vi "SCA-RT_old.vi"() -> ()   [LabVIEW 2016]
uses:
  <vilib>/Platform/TimedLoop/XDataNode/wakeup.ctl
  <vilib>/Platform/TimedLoop/XDataNode/XDNodeRunTimeDep.lvlib
  <vilib>/Platform/TimedLoop/XDataNode/nitl_modes.ctl
  <vilib>/Platform/TimedLoop/XDataNode/timing_clust.ctl
  <vilib>/Platform/TimedLoop/XDataNode/XDataNode.xnode
  <vilib>/Motion/BlockNode/FB.NIMotion.xnode
  <vilib>/Platform/TimedLoop/XDataNode/loadnilvce.vi
  Users/wymanm/Desktop/Sample Changer - Copy/controls/state control sample changer.ctl
  <vilib>/Instr/_visa.llb/VISA Configure Serial Port (Instr).vi
  <vilib>/Analysis/NI_AALBase.lvlib
  <vilib>/Analysis/baseanly.llb/Mean (DBL).vi
  controls/SCA states.ctl
  controls/Encoder bit cluster.ctl
  Common-Control/Gate Valve Readback.ctl
  Common-Control/Horizontal Rod states.ctl
  controls/Vertical Rod states.ctl
  <vilib>/NI_Real-Time Target Support.lvlib
  <vilib>/Motion/Express/_s/nimc.fb.straightLineMove.startStraightLineMove.axis.modeRelative.0.vi
  Common-Control/GP307 cluster.ctl
panel:
  in  "Sample Rod Min Count":u32
  in  "Sample Rod Max Count":u32
  in  "Insert Rod Max Count":u32
  in  "Insert Rod Min Count":u32
  in  "Retract Rod Min Count":u32
  in  "Retract Rod Max Count":u32
  out "Encoder loop error":errorcluster
  out "Convectron readback loop error":errorcluster
  out "HV Control loop error":errorcluster
  out "Rotate Wheel error":errorcluster
  out "Ion Source Vac Cluster":T1
  out "Bellows Vac Cluster":T1
  in  "Wheel GV Min Count":i32
  out "Start Sample Change":bool
  out "SCA-cRIO error":errorcluster
  in  "Rollover Sample":i8=54
  out "Insert Rod Status":T2
  out "Retract Rod Status":T2
  out "Sample Rod status":T3
  out "Wheel GV":T4
  out "Raw bits":bool[](array[boolean])
  out "Converted bits":bool[](array[boolean])
  out "Immersion Lens I read":dbl format="%0.2f"
  out "Immersion Lens V read":dbl format="%0.2f"
  out "SCA next state":T5
  out "Extractor I read":dbl
  out "Extractor V read":dbl
  out "Extractor V set":dbl
  out "Cathode V read":dbl
  out "Cathode I read":dbl
  out "Cathode V set":dbl
  in  "Execute Move":bool
  out "New Move":dbl
  out "Encoder Destination":dbl
  in  "Step Window Radius":i16=2
  out "In Range?":bool
  out "Window Limit 2":u32
  out "Window Limit 1":u32
  out "Encoder position":u16
  out "change sample start end":bool
  out "start sample change":bool
  in  "clear error 3":bool
  in  "clear error 2":bool
  out "set cold cathode on 2":bool
  out "Rotate Wheel":bool
  out "Venting Source":bool
  out "Pumping out Source":bool
  out "insert Retract Rod":bool
  out "retract Retract Rod":bool
  out "Open Wheel GV":bool
  out "Close Wheel GV":bool
  out "insert Insert Rod":bool
  out "retract Insert Rod":bool
  out "insert Sample Rod":bool
  out "retract Sample Rod":bool
  in  "clear error":bool
  out "action":string
  out "Vac Readback Loop error":errorcluster
  out "Sample Wheel Convectron":string
  out "Sample Rod UP sensor":bool
  out "Sample Rod DOWN sensor":bool
  out "done":bool
  out "Insert Rod IN sensor":bool
  out "Insert Rod OUT sensor":bool
  out "Retract Rod IN sensor":bool
  out "Retract Rod OUT sensor":bool
  out "Sensor loop error":errorcluster
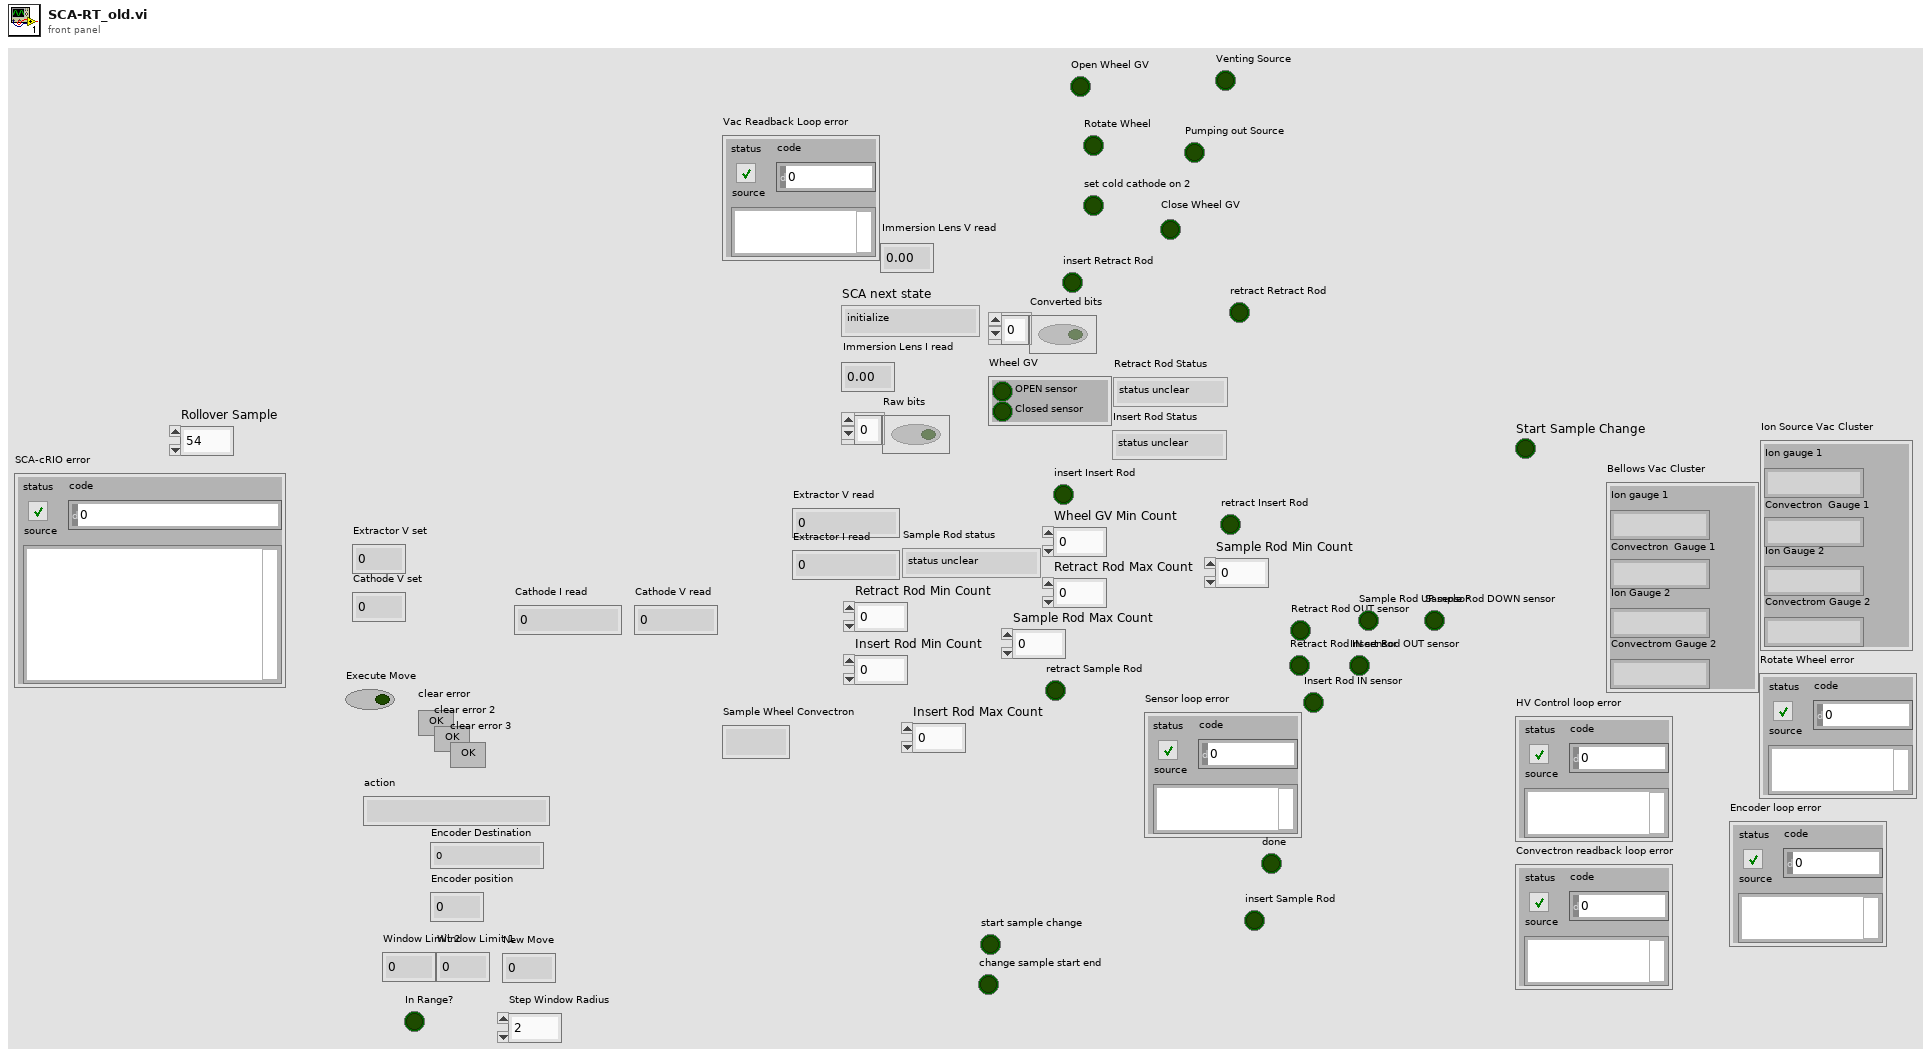
[diagram p1: front panel]
types:
  T1 = typedef "GP307 cluster.ctl" = cluster{"Ion gauge 1":string, "Convectron  Gauge 1 ":string, "Ion Gauge 2":string, "Convectrom Gauge 2":string}
  T2 = typedef "Horizontal Rod states.ctl" = enum16{"status unclear", "rod in", "rod out"}
  T3 = typedef "Vertical Rod states.ctl" = enum16{"status unclear", "rod down", "rod up"}
  T4 = typedef "Gate Valve Readback.ctl" = cluster{"OPEN sensor":bool, "Closed sensor":bool}
  T5 = typedef "SCA states.ctl" = enum16{"initialize", "wait", "change sample start", "change sample", "check position", "wait position", "rotate wheel", "sample change complete", "sample rod up", "sample rod down", "retract rod in", "retract rod out", "insert rod in", "insert rod out", "wheel GV open", "wheel GV close", "vent source", "pump source"}
  T6 = typedef "GV states.ctl" = enum16{"status unclear", "closed", "open"}
  T7 = typedef "XDNodeRunTimeDep.lvlib/timing_clust.ctl" = cluster{"Expected End [f-1]":u64, "Actual End [f-1]":u64, "Finished Late? [f-1]":bool, "Expected End [i-1]":u64, "Actual End [i-1]":u64, "Finished Late? [i-1]":bool, "Expected Start [i]":u64, "Actual Start [i]":u64, "Expected Start [f]":u64, "Actual Start [f]":u64, "Source Name":string, "Structure Name":string, "Period":i64, "Deadline":i64, "Offset":i64, "Start":i64, "Priority":i32, "Timeout":i32, "Mode":T8, "Wakeup Reason":T9, "Error":errorcluster, "Source Type":string, "Secondary Source Type":string, "Global End Time":u64, "Global Start Time":u64, "Frame Duration":u64, "Iteration Duration":u64, "Assigned CPU":i32, "I/O Scan Engine Mode":u32}
  T8 = typedef "XDNodeRunTimeDep.lvlib/nitl_modes.ctl" = enum32{"No Change", "Process missed periods, maintain original phase", "Discard missed periods, maintain original phase", "Process missed periods, ignore original phase", "Discard missed periods, ignore original phase"}
  T9 = typedef "XDNodeRunTimeDep.lvlib/wakeup.ctl" = enum32{"Normal", "Aborted", "Asynchronous wakeup", "Timing source error", "Timed loop error", "Timeout"}
  T10 = typedef "Encoder bit cluster.ctl" = cluster{"MSB":bool, "13th bit":bool, "12th bit":bool, "11th bit":bool, "10th bit":bool, "9th bit":bool, "8th bit":bool, "7th bit":bool, "6th bit":bool, "5th bit":bool, "4th bit":bool, "3rd bit":bool, "2nd bit":bool, "LSB":bool}
  T11 = typedef "state control sample changer.ctl" = string
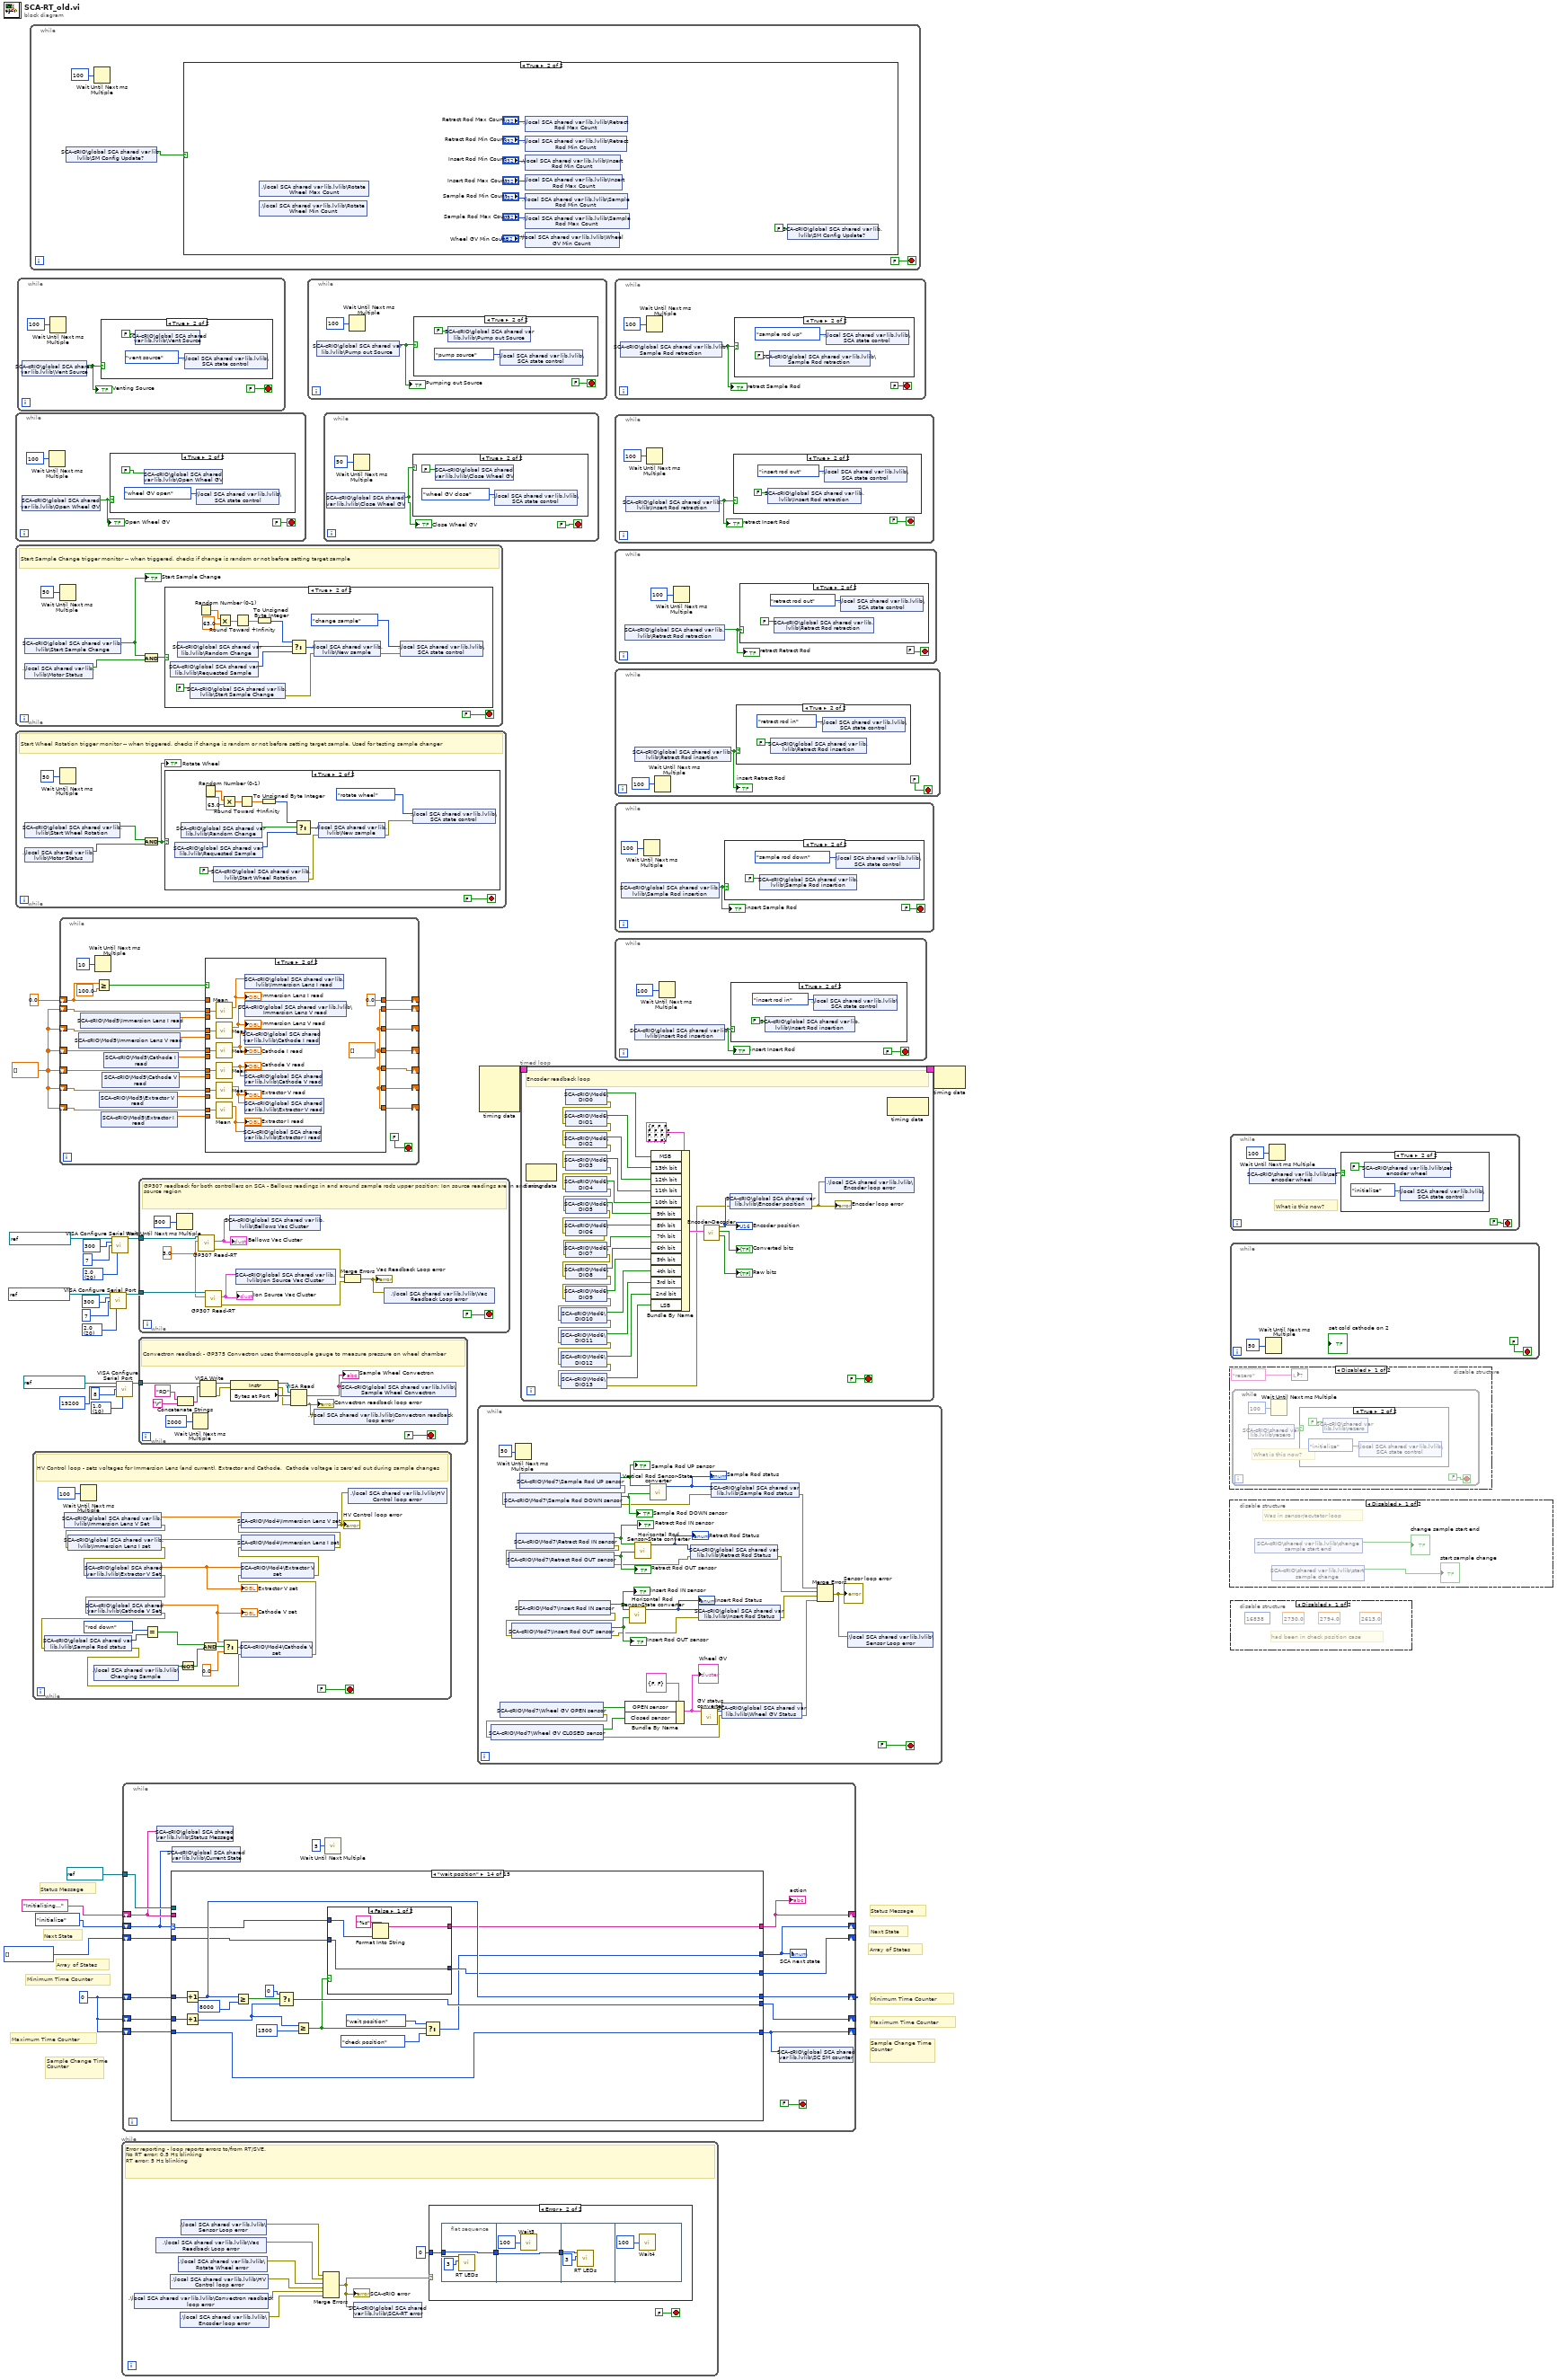
[diagram p0: block diagram]
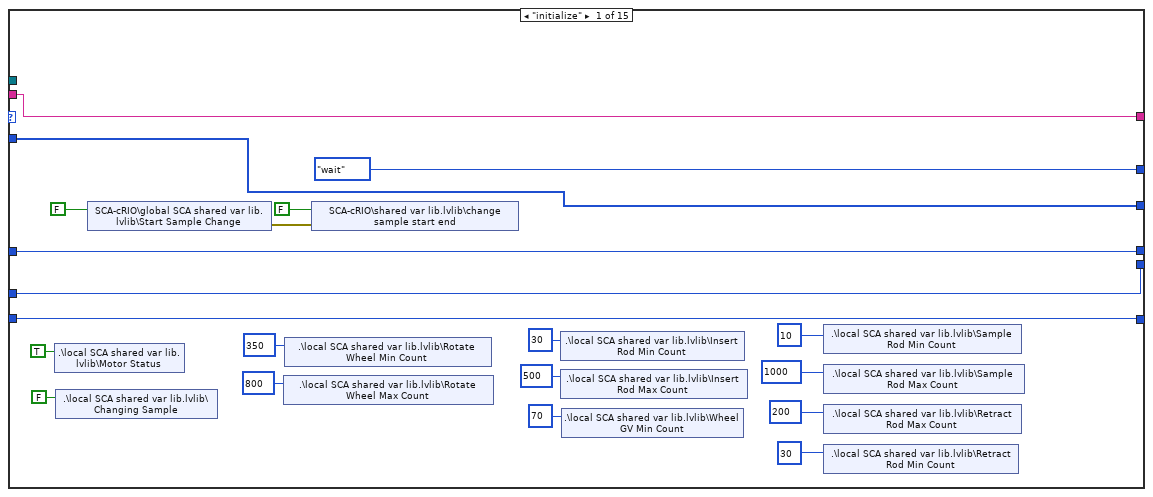
[diagram p5: hidden frame]
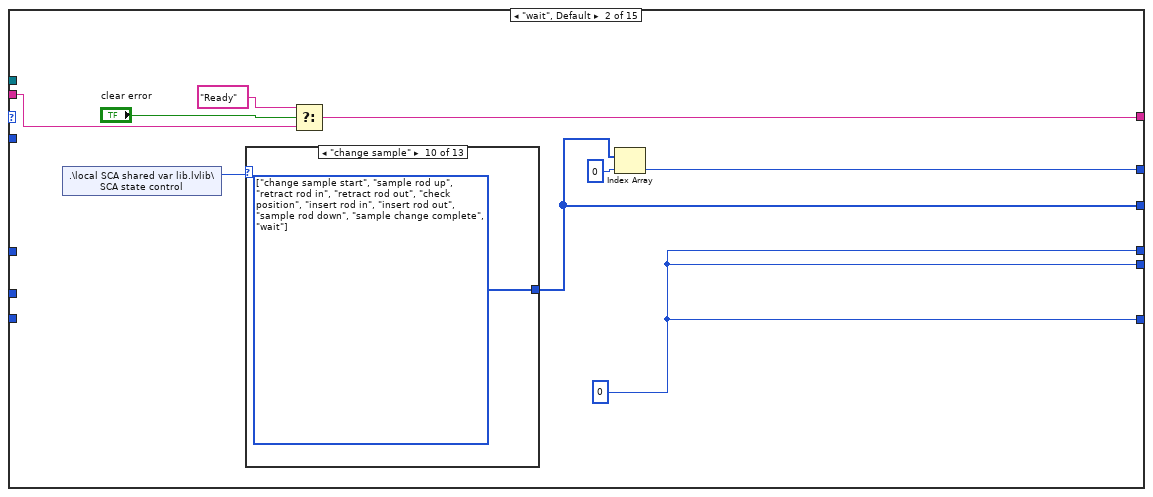
[diagram p6: hidden frame]
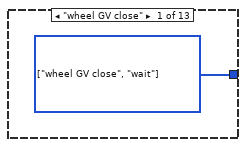
[diagram p7: hidden frame]
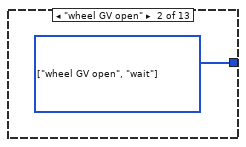
[diagram p8: hidden frame]
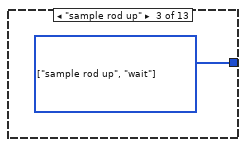
[diagram p9: hidden frame]
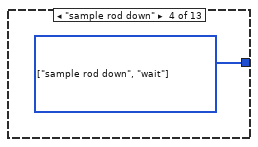
[diagram p10: hidden frame]
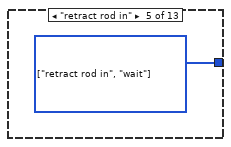
[diagram p11: hidden frame]
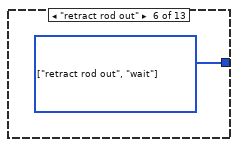
[diagram p12: hidden frame]
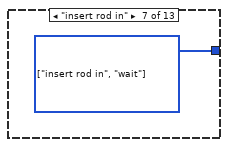
[diagram p13: hidden frame]
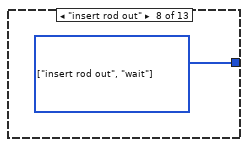
[diagram p14: hidden frame]
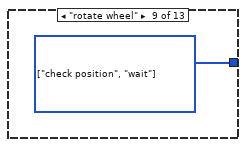
[diagram p15: hidden frame]
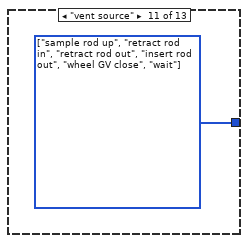
[diagram p16: hidden frame]
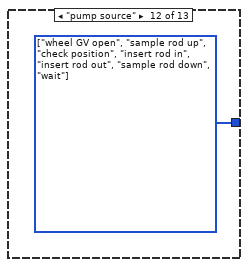
[diagram p17: hidden frame]
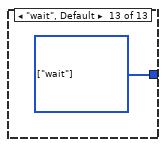
[diagram p18: hidden frame]
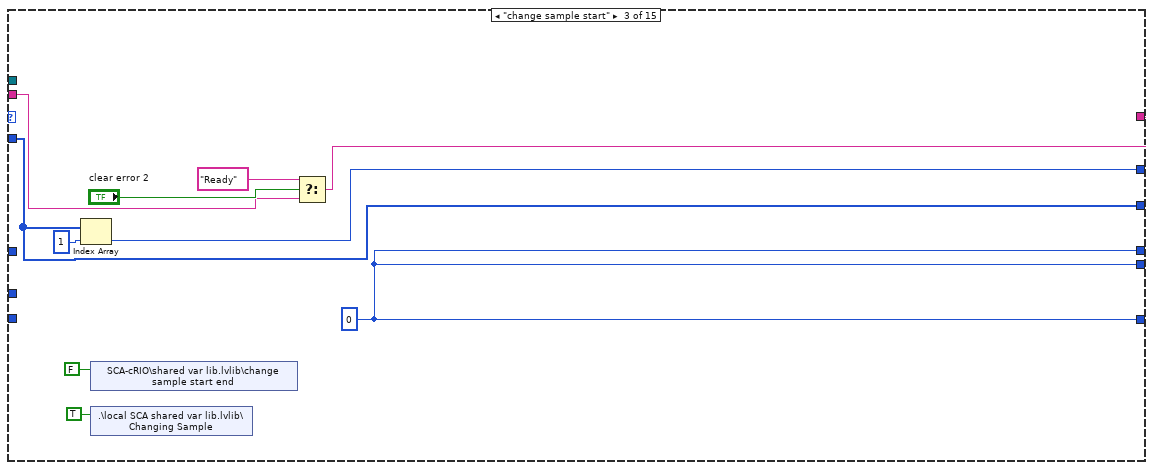
[diagram p19: hidden frame]
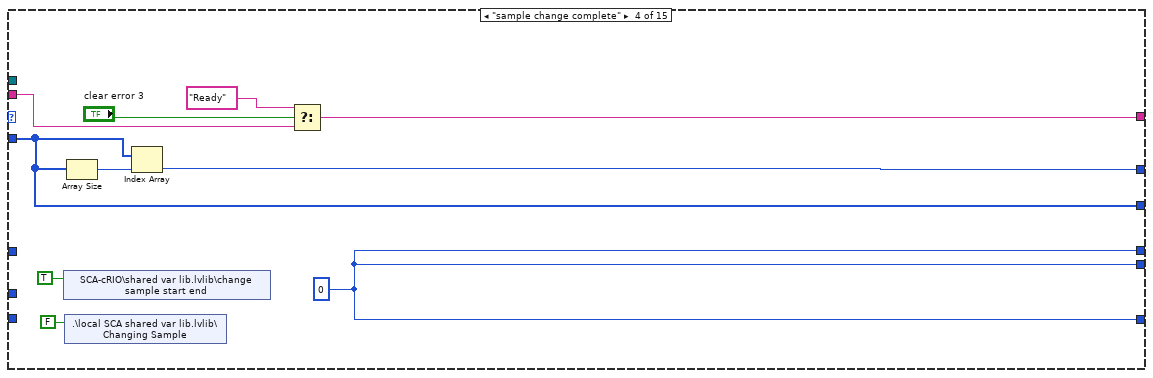
[diagram p20: hidden frame]
diagram:
  w2 = dbl[] []
  w19 = u16 20 items=["1.0"=10, "1.5"=15, "2.0"=20] ("stop bits (10: 1 bit)")
  w23 = u16 10 items=["1.0"=10, "1.5"=15, "2.0"=20] ("stop bits (10: 1 bit)")
  w13 = u16 20 items=["1.0"=10, "1.5"=15, "2.0"=20] ("stop bits (10: 1 bit)")
  w7 = u32 0
  w24 = T5[] [] items=["initialize", "wait", "change sample start", "change sample", "check position", "wait position", "rotate wheel", "sample change complete", "sample rod up", "sample rod down", "retract rod in", "retract rod out", "insert rod in", "insert rod out", "wheel GV open", "wheel GV close", "vent source", "pump source"]
  # "Status Message"
  # "Array of States"
  # "Next State"
  # "Sample Change Time Counter"
  # "Maximum Time Counter"
  # "Minimum Time Counter"
  # "Status Message"
  # "Array of States"
  # "Next State"
  # "Sample Change Time Counter"
  # "Maximum Time Counter"
  # "Minimum Time Counter"
  n1 = while {
    stop <- FALSE stop-if-true
    n2 = shared-variable "SCA-cRIO\\global SCA shared var lib.lvlib\\Open Wheel GV"() -> (w26:bool)  [unwired: 1 in, 1 out]
    "Open Wheel GV" <- w26
    n3 = Wait Until Next ms Multiple(millisecond multiple=u32 100) -> ()  [unwired: 1 out]
    n4 = case shown="True" w26 {
      frame False {
      }
      frame True {
        n5 = shared-variable "SCA-cRIO\\global SCA shared var lib.lvlib\\Open Wheel GV"(FALSE ("rod up shared")) -> ()  [unwired: 1 in, 1 out]
        n6 = shared-variable ".\\local SCA shared var lib.lvlib\\SCA state control"(SCA_states."wheel GV open" ("SC2 state")) -> ()  [unwired: 1 in, 1 out]
      }
    }
  }
  n7 = while {
    stop <- FALSE stop-if-true
    # "Start Sample Change trigger monitor -- when triggered, checks if change is random or not before setting target sample"
    n8 = shared-variable "SCA-cRIO\\global SCA shared var lib.lvlib\\Start Sample Change"() -> (w32:bool)  [unwired: 1 in, 1 out]
    "Start Sample Change" <- w32
    n9 = shared-variable ".\\local SCA shared var lib.lvlib\\Motor Status"() -> (w30:bool)  [unwired: 1 in, 1 out]
    n10 = Wait Until Next ms Multiple(millisecond multiple=u32 50) -> ()  [unwired: 1 out]
    n11 = And(x=w32, y=w30) -> (x .and. y?=w31:bool)
    n12 = case shown="True" w31 {
      frame False {
      }
      frame True {
        n13 = shared-variable "SCA-cRIO\\global SCA shared var lib.lvlib\\Requested Sample"() -> (w38:u8)  [unwired: 1 in, 1 out]
        n14 = shared-variable "SCA-cRIO\\global SCA shared var lib.lvlib\\Random Change"() -> (w37:bool)  [unwired: 1 in, 1 out]
        n15 = shared-variable "SCA-cRIO\\global SCA shared var lib.lvlib\\Start Sample Change"(FALSE ("rod up shared")) -> (error out=w35:errorcluster)  [unwired: 1 in]
        n16 = Random Number (0-1)() -> (number: 0 to 1=w42:dbl)
        n17 = Multiply(x=w42, y=63.0) -> (x*y=w40:dbl)
        n18 = Round Toward +Infinity(x=w40) -> (ceil(x): smallest int >= x=w43:dbl)
        n19 = To Unsigned Byte Integer(number=w43) -> (unsigned 8bit integer=w44:u8)
        n20 = Select(t=w44, s=w37, f=w38) -> (s? t:f=w39:u8)
        n21 = shared-variable ".\\local SCA shared var lib.lvlib\\New sample"(w39, error in=w35) -> (error out=w36:errorcluster)
        n22 = shared-variable ".\\local SCA shared var lib.lvlib\\SCA state control"(SCA_states."change sample" ("SC2 state"), error in=w36) -> ()  [unwired: 1 out]
      }
    }
  }
  n23 = while {
    stop <- FALSE stop-if-true
    # "Start Wheel Rotation trigger monitor -- when triggered, checks if change is random or not before setting target sample. Used for testing sample changer"
    n24 = shared-variable "SCA-cRIO\\global SCA shared var lib.lvlib\\Start Wheel Rotation"() -> (w49:bool)  [unwired: 1 in, 1 out]
    n25 = shared-variable ".\\local SCA shared var lib.lvlib\\Motor Status"() -> (w48:bool)  [unwired: 1 in, 1 out]
    n26 = Wait Until Next ms Multiple(millisecond multiple=u32 50) -> ()  [unwired: 1 out]
    n27 = And(x=w49, y=w48) -> (x .and. y?=w47:bool)
    "Rotate Wheel" <- w47
    n28 = case shown="True" w47 {
      frame False {
      }
      frame True {
        n29 = shared-variable "SCA-cRIO\\global SCA shared var lib.lvlib\\Requested Sample"() -> (w55:u8)  [unwired: 1 in, 1 out]
        n30 = shared-variable "SCA-cRIO\\global SCA shared var lib.lvlib\\Random Change"() -> (w54:bool)  [unwired: 1 in, 1 out]
        n31 = Random Number (0-1)() -> (number: 0 to 1=w59:dbl)
        n32 = shared-variable "SCA-cRIO\\global SCA shared var lib.lvlib\\Start Wheel Rotation"(FALSE ("rod up shared")) -> (error out=w52:errorcluster)  [unwired: 1 in]
        n33 = Multiply(x=w59, y=63.0) -> (x*y=w57:dbl)
        n34 = Round Toward +Infinity(x=w57) -> (ceil(x): smallest int >= x=w60:dbl)
        n35 = To Unsigned Byte Integer(number=w60) -> (unsigned 8bit integer=w61:u8)
        n36 = Select(t=w61, s=w54, f=w55) -> (s? t:f=w56:u8)
        n37 = shared-variable ".\\local SCA shared var lib.lvlib\\New sample"(w56, error in=w52) -> (error out=w53:errorcluster)
        n38 = shared-variable ".\\local SCA shared var lib.lvlib\\SCA state control"(SCA_states."rotate wheel" ("SC2 state"), error in=w53) -> ()  [unwired: 1 out]
      }
    }
  }
  n39 = while {
    stop <- FALSE stop-if-true
    n40 = shared-variable "SCA-cRIO\\global SCA shared var lib.lvlib\\Vent Source"() -> (w65:bool)  [unwired: 1 in, 1 out]
    "Venting Source" <- w65
    n41 = Wait Until Next ms Multiple(millisecond multiple=u32 100) -> ()  [unwired: 1 out]
    n42 = case shown="True" w65 {
      frame False {
      }
      frame True {
        n43 = shared-variable "SCA-cRIO\\global SCA shared var lib.lvlib\\Vent Source"(FALSE ("rod up shared")) -> ()  [unwired: 1 in, 1 out]
        n44 = shared-variable ".\\local SCA shared var lib.lvlib\\SCA state control"(SCA_states."vent source" ("SC2 state")) -> ()  [unwired: 1 in, 1 out]
      }
    }
  }
  n45 = while {
    stop <- FALSE stop-if-true
    n46 = shared-variable "SCA-cRIO\\global SCA shared var lib.lvlib\\SM Config Update?"() -> (w71:bool)  [unwired: 1 in, 1 out]
    n47 = Wait Until Next ms Multiple(millisecond multiple=u32 100) -> ()  [unwired: 1 out]
    n48 = case shown="True" w71 {
      frame False {
      }
      frame True {
        n49 = shared-variable ".\\local SCA shared var lib.lvlib\\Rotate Wheel Min Count"() -> ()  [unwired: 2 in, 1 out]
        n50 = shared-variable ".\\local SCA shared var lib.lvlib\\Rotate Wheel Max Count"() -> ()  [unwired: 2 in, 1 out]
        n51 = shared-variable ".\\local SCA shared var lib.lvlib\\Retract Rod Max Count"("Retract Rod Max Count") -> ()  [unwired: 1 in, 1 out]
        n52 = shared-variable ".\\local SCA shared var lib.lvlib\\Retract Rod Min Count"("Retract Rod Min Count") -> ()  [unwired: 1 in, 1 out]
        n53 = shared-variable ".\\local SCA shared var lib.lvlib\\Insert Rod Min Count"("Insert Rod Min Count") -> ()  [unwired: 1 in, 1 out]
        n54 = shared-variable ".\\local SCA shared var lib.lvlib\\Insert Rod Max Count"("Insert Rod Max Count") -> ()  [unwired: 1 in, 1 out]
        n55 = shared-variable ".\\local SCA shared var lib.lvlib\\Sample Rod Min Count"("Sample Rod Min Count") -> ()  [unwired: 1 in, 1 out]
        n56 = shared-variable ".\\local SCA shared var lib.lvlib\\Sample Rod Max Count"("Sample Rod Max Count") -> ()  [unwired: 1 in, 1 out]
        n57 = shared-variable ".\\local SCA shared var lib.lvlib\\Wheel GV Min Count"("Wheel GV Min Count") -> ()  [unwired: 1 in, 1 out]
        n58 = shared-variable "SCA-cRIO\\global SCA shared var lib.lvlib\\SM Config Update?"(FALSE ("SM Config Update?")) -> ()  [unwired: 1 in, 1 out]
      }
    }
  }
  n59 = while {
    stop <- FALSE stop-if-true
    # "HV Control loop - sets voltages for Immersion Lens (and current), Extractor and Cathode.  Cathode voltage is zero'ed out during sample changes"
    n60 = shared-variable "SCA-cRIO\\global SCA shared var lib.lvlib\\Immersion Lens V Set"() -> (w94:dbl, error out=w92:errorcluster)  [unwired: 1 in]
    n61 = shared-variable "SCA-cRIO\\global SCA shared var lib.lvlib\\Immersion Lens I set"(error in=w92) -> (w93:dbl, error out=w91:errorcluster)
    n62 = Wait Until Next ms Multiple(millisecond multiple=u32 100) -> ()  [unwired: 1 out]
    n63 = shared-variable "SCA-cRIO\\global SCA shared var lib.lvlib\\Extractor V Set"(error in=w91) -> (w100:dbl, error out=w90:errorcluster)
    "Extractor V set" <- w100
    n64 = shared-variable "SCA-cRIO\\global SCA shared var lib.lvlib\\Cathode V Set"(error in=w90) -> (w97:dbl, error out=w89:errorcluster)
    "Cathode V set" <- w97
    n65 = shared-variable "SCA-cRIO\\global SCA shared var lib.lvlib\\Sample Rod status"(error in=w89) -> (w83:T3, error out=w81:errorcluster)
    n66 = shared-variable ".\\local SCA shared var lib.lvlib\\Changing Sample"() -> (w99:bool)  [unwired: 1 in, 1 out]
    n67 = Equal?(x=Vertical_Rod_states."rod down", y=w83) -> (x = y?=w84:bool)
    n68 = Not(x=w99) -> (.not. x?=w80:bool)
    n69 = And(x=w84, y=w80) -> (x .and. y?=w98:bool)
    n70 = Select(t=w97, s=w98, f=0.0) -> (s? t:f=w95:dbl)
    n71 = shared-variable "SCA-cRIO\\Mod4\\Cathode V set"(w95, error in=w81) -> (error out=w86:errorcluster)
    n72 = shared-variable "SCA-cRIO\\Mod4\\Extractor V set"(w100, error in=w86) -> (error out=w87:errorcluster)
    n73 = shared-variable "SCA-cRIO\\Mod4\\Immersion Lens I set"(w93, error in=w87) -> (error out=w88:errorcluster)
    n74 = shared-variable "SCA-cRIO\\Mod4\\Immersion Lens V set"(w94, error in=w88) -> (error out=w85:errorcluster)
    "HV Control loop error" <- w85
    n75 = shared-variable ".\\local SCA shared var lib.lvlib\\HV Control loop error"(w85) -> ()  [unwired: 1 in, 1 out]
  }
  n76 = while {
    shift-right: [w119] -> _
    shift-left: 0.0 ("AI1") -> [w122]
    shift-right: [w117] -> _
    shift-left: w2 -> [w116]
    shift-right: [w118] -> _
    shift-left: w2 -> [w115]
    shift-right: [w113] -> _
    shift-left: w2 -> [w112]
    shift-right: [w110] -> _
    shift-left: w2 -> [w109]
    shift-right: [w104] -> _
    shift-left: w2 -> [w107]
    shift-right: [w103] -> _
    shift-left: w2 -> [w108]
    stop <- FALSE stop-if-true
    n77 = shared-variable "SCA-cRIO\\Mod5\\Immersion Lens V read"() -> (w105:dbl)  [unwired: 1 in, 1 out]
    n78 = shared-variable "SCA-cRIO\\Mod5\\Immersion Lens I read"() -> (w106:dbl)  [unwired: 1 in, 1 out]
    n79 = Wait Until Next ms Multiple(millisecond multiple=u32 10) -> ()  [unwired: 1 out]
    n80 = Greater Or Equal?(x=w122, y=100.0) -> (x >= y?=w120:bool)
    n81 = shared-variable "SCA-cRIO\\Mod5\\Extractor V read"() -> (w114:dbl)  [unwired: 1 in, 1 out]
    n82 = shared-variable "SCA-cRIO\\Mod5\\Extractor I read"() -> (w111:dbl)  [unwired: 1 in, 1 out]
    n83 = shared-variable "SCA-cRIO\\Mod5\\Cathode V read"() -> (w124:dbl)  [unwired: 1 in, 1 out]
    n84 = shared-variable "SCA-cRIO\\Mod5\\Cathode I read"() -> (w123:dbl)  [unwired: 1 in, 1 out]
    n85 = case shown="True" w120 {
      tunnel: w124 -> [w142 _]
      tunnel: w123 -> [w143 _]
      tunnel: w122 -> [w146 _]
      tunnel: [w145 0.0 ("AI1")] -> w119
      tunnel: [w144 w150] -> w118
      tunnel: [w141 w150] -> w117
      tunnel: w116 -> [w140 w158]
      tunnel: w115 -> [w139 w159]
      tunnel: w114 -> [w138 _]
      tunnel: [w137 w150] -> w113
      tunnel: w112 -> [w136 w157]
      tunnel: w111 -> [w135 _]
      tunnel: [w134 w150] -> w110
      tunnel: w109 -> [w133 w156]
      tunnel: w108 -> [w132 w149]
      tunnel: w107 -> [w131 w148]
      tunnel: w106 -> [w130 _]
      tunnel: w105 -> [w129 _]
      tunnel: [w128 w150] -> w104
      tunnel: [w127 w150] -> w103
      frame False {
        n86 = Build Array (concatenate)(w130, w131) -> (w128:dbl[])
        n87 = Build Array (concatenate)(w129, w132) -> (w127:dbl[])
        n88 = Build Array (concatenate)(w143, w139) -> (w144:dbl[])
        n89 = Build Array (concatenate)(w142, w140) -> (w141:dbl[])
        n90 = Build Array (concatenate)(w138, w136) -> (w137:dbl[])
        n91 = Build Array (concatenate)(w135, w133) -> (w134:dbl[])
        n92 = Increment(x=w146) -> (x+1=w145:dbl)
      }
      frame True {
        w150 = dbl[] []
        n93 = call-poly <vilib>:"Mean.vi"("X"=w148) -> ("mean"=w147:dbl)  [unwired: 1 out]
        "Immersion Lens I read" <- w147
        n94 = call-poly <vilib>:"Mean.vi"("X"=w149) -> ("mean"=w151:dbl)  [unwired: 1 out]
        "Immersion Lens V read" <- w151
        n95 = call-poly <vilib>:"Mean.vi"("X"=w159) -> ("mean"=w155:dbl)  [unwired: 1 out]
        "Cathode I read" <- w155
        n96 = call-poly <vilib>:"Mean.vi"("X"=w158) -> ("mean"=w154:dbl)  [unwired: 1 out]
        "Cathode V read" <- w154
        n97 = call-poly <vilib>:"Mean.vi"("X"=w157) -> ("mean"=w153:dbl)  [unwired: 1 out]
        "Extractor V read" <- w153
        n98 = call-poly <vilib>:"Mean.vi"("X"=w156) -> ("mean"=w152:dbl)  [unwired: 1 out]
        "Extractor I read" <- w152
        n99 = shared-variable "SCA-cRIO\\global SCA shared var lib.lvlib\\Immersion Lens I read"(w147) -> ()  [unwired: 1 in, 1 out]
        n100 = shared-variable "SCA-cRIO\\global SCA shared var lib.lvlib\\Immersion Lens V read"(w151) -> ()  [unwired: 1 in, 1 out]
        n101 = shared-variable "SCA-cRIO\\global SCA shared var lib.lvlib\\Cathode I read"(w155) -> ()  [unwired: 1 in, 1 out]
        n102 = shared-variable "SCA-cRIO\\global SCA shared var lib.lvlib\\Cathode V read"(w154) -> ()  [unwired: 1 in, 1 out]
        n103 = shared-variable "SCA-cRIO\\global SCA shared var lib.lvlib\\Extractor V read"(w153) -> ()  [unwired: 1 in, 1 out]
        n104 = shared-variable "SCA-cRIO\\global SCA shared var lib.lvlib\\Extractor I read"(w152) -> ()  [unwired: 1 in, 1 out]
      }
    }
  }
  n105 = call-poly "VISA Configure Serial Port"("VISA resource name"=refnum<visa-resource-name> "ASRL6::INSTR", "baud rate (9600)"=u32 300, "data bits (8)"=u16 7, "stop bits (10: 1 bit)"=w13) -> ("VISA resource name out"=w14:refnum<visa-resource-name>)  [unwired: 10 in, 1 out]
  n106 = call-poly "VISA Configure Serial Port"("VISA resource name"=refnum<visa-resource-name> "ASRL8::INSTR", "baud rate (9600)"=u32 300, "data bits (8)"=u16 7, "stop bits (10: 1 bit)"=w19) -> ("VISA resource name out"=w20:refnum<visa-resource-name>)  [unwired: 10 in, 1 out]
  n107 = call-poly "VISA Configure Serial Port"("VISA resource name"=refnum<visa-resource-name> "ASRL7::INSTR", "baud rate (9600)"=u32 19200, "data bits (8)"=u16 8, "stop bits (10: 1 bit)"=w23) -> ("VISA resource name out"=w9:refnum<visa-resource-name>)  [unwired: 10 in, 1 out]
  n108 = while {
    stop <- FALSE stop-if-true
    # "Error reporting - loop reports errors to/from RT/SVE. \nNo RT error: 0.5 Hz blinking\nRT error: 5 Hz blinking"
    n109 = shared-variable ".\\local SCA shared var lib.lvlib\\Convectron readback loop error"() -> (w162:errorcluster)  [unwired: 1 in, 1 out]
    n110 = shared-variable ".\\local SCA shared var lib.lvlib\\Vac Readback Loop error"() -> (w167:errorcluster)  [unwired: 1 in, 1 out]
    n111 = shared-variable ".\\local SCA shared var lib.lvlib\\HV Control loop error"() -> (w163:errorcluster)  [unwired: 1 in, 1 out]
    n112 = shared-variable ".\\local SCA shared var lib.lvlib\\Rotate Wheel error"() -> (w164:errorcluster)  [unwired: 1 in, 1 out]
    n113 = shared-variable ".\\local SCA shared var lib.lvlib\\Encoder loop error"() -> (w161:errorcluster)  [unwired: 1 in, 1 out]
    n114 = shared-variable ".\\local SCA shared var lib.lvlib\\Sensor Loop error"() -> (w168:errorcluster)  [unwired: 1 in, 1 out]
    n115 = Merge Errors(w168, w167, w164, w163, w162, w161) -> (w166:errorcluster)
    "SCA-cRIO error" <- w166
    n116 = shared-variable "SCA-cRIO\\global SCA shared var lib.lvlib\\SCA-RT error"(w166) -> ()  [unwired: 1 in, 1 out]
    n117 = case shown="Error" w166 {
      tunnel: 0 -> [w172 w180]
      frame No Error {
        n118 = flat-sequence {
          tunnel: w172 -> [w173]
          tunnel: [w173] -> w170
          tunnel: [w175] -> w171
          tunnel: w170 -> [w175]
          tunnel: w171 -> [w177]
          frame #0 {
            n119 = call <vilib>:"RT LEDs.vi"("State"=3, "LED Num"=w173) -> ()  [unwired: 4 in, 2 out]
          }
          frame #1 {
            n120 = call "Wait"("Count(mSec)"=u16 1000) -> ()  [unwired: 1 out]
          }
          frame #2 {
            n121 = call <vilib>:"RT LEDs.vi"("State"=3, "LED Num"=w177) -> ()  [unwired: 4 in, 2 out]
          }
          frame #3 {
            n122 = call "Wait2"("Count(mSec)"=u16 1000) -> ()  [unwired: 1 out]
          }
        }
      }
      frame Error {
        n123 = flat-sequence {
          tunnel: [w183] -> w182
          tunnel: w180 -> [w183]
          tunnel: w182 -> [w185]
          tunnel: [w185] -> w181
          tunnel: w181 -> [w187]
          frame #0 {
            n124 = call <vilib>:"RT LEDs.vi"("State"=3, "LED Num"=w183) -> ()  [unwired: 4 in, 2 out]
          }
          frame #1 {
            n125 = call "Wait3"("Count(mSec)"=u16 100) -> ()  [unwired: 1 out]
          }
          frame #2 {
            n126 = call <vilib>:"RT LEDs.vi"("State"=3, "LED Num"=w187) -> ()  [unwired: 4 in, 2 out]
          }
          frame #3 {
            n127 = call "Wait4"("Count(mSec)"=u16 100) -> ()  [unwired: 1 out]
          }
        }
      }
    }
  }
  n128 = while {
    shift-right: [w202] -> _
    shift-left: SCA_states."initialize" ("SC2 state") -> [w192]
    shift-right: [w191] -> _
    shift-left: w24 -> [w201]
    shift-right: [w199] -> _
    shift-left: w7 -> [w200]
    shift-right: [w198] -> _
    shift-left: "Initializing..." -> [w193]
    shift-right: [w196] -> _
    shift-left: w7 -> [w197]
    shift-right: [w194] -> _
    shift-left: w7 -> [w195]
    tunnel: refnum<k21> "Axis 1" ("resource") -> [w203]
    stop <- FALSE ("stop 2") stop-if-true
    n129 = shared-variable "SCA-cRIO\\global SCA shared var lib.lvlib\\Status Message"(w193) -> ()  [unwired: 1 in, 1 out]
    n130 = case shown="\"wait position\"" w192 {
      selector: w192 -> [_ _ _ _ w275 w293 w316 w350 w384 w418 w452 w486 w522 w576 w607]
      tunnel: w203 -> [_ _ _ _ _ _ _ _ _ _ _ _ w537 _ _]
      tunnel: [SCA_states."wait" ("SC2 state") w226 w256 w266 w280 w299 w324 w358 w392 w426 w460 w494 w531 w578 w617] -> w202
      tunnel: w201 -> [w216 _ w248 w258 w276 w294 w317 w351 w385 w419 w453 w487 w523 w575 w606]
      tunnel: w200 -> [w219 _ _ _ w283 w302 w330 w364 w398 w432 w466 w500 w535 w588 w612]
      tunnel: [w219 w229 w251 w261 w282 w301 w310 w344 w379 w413 w447 w481 w518 w589 w612] -> w199
      tunnel: [w216 w227 w248 w258 w276 w294 w319 w353 w387 w421 w455 w489 w532 w585 w606] -> w191
      tunnel: w193 -> [w217 w232 w254 w264 _ _ _ _ _ _ _ _ _ _ _]
      tunnel: [w217 w231 w253 w263 w279 w298 w326 w360 w394 w428 w462 w496 w530 w584 w616] -> w198
      tunnel: w197 -> [w220 _ _ _ w281 w300 w323 w357 w391 w425 w459 w493 w533 w586 _]
      tunnel: [w220 w229 w251 w261 w268 w297 w321 w355 w389 w423 w457 w491 w526 w580 u32 0 ("t")] -> w196
      tunnel: w195 -> [w221 _ _ _ w278 w296 w320 w354 w388 w422 w456 w490 w517 w572 w615]
      tunnel: [w221 w229 w251 w261 w278 w296 w320 w354 w388 w422 w456 w490 w517 w572 w615] -> w194
      frame "initialize" {
        n131 = shared-variable ".\\local SCA shared var lib.lvlib\\Motor Status"(TRUE ("Motor Status")) -> ()  [unwired: 1 in, 1 out]
        n132 = shared-variable ".\\local SCA shared var lib.lvlib\\Changing Sample"(FALSE ("Changing Sample")) -> ()  [unwired: 1 in, 1 out]
        n133 = shared-variable "SCA-cRIO\\global SCA shared var lib.lvlib\\Start Sample Change"(FALSE ("start sample change")) -> (error out=w224:errorcluster)  [unwired: 1 in]
        n134 = shared-variable ".\\local SCA shared var lib.lvlib\\Rotate Wheel Max Count"(u32 800 ("Rotate Wheel Max Count")) -> ()  [unwired: 1 in, 1 out]
        n135 = shared-variable ".\\local SCA shared var lib.lvlib\\Rotate Wheel Min Count"(u32 350 ("Rotate Wheel Min Count")) -> ()  [unwired: 1 in, 1 out]
        n136 = shared-variable "SCA-cRIO\\shared var lib.lvlib\\change sample start end"(FALSE ("change sample start end"), error in=w224) -> ()  [unwired: 1 out]
        n137 = shared-variable ".\\local SCA shared var lib.lvlib\\Insert Rod Min Count"(u32 30 ("y")) -> ()  [unwired: 1 in, 1 out]
        n138 = shared-variable ".\\local SCA shared var lib.lvlib\\Insert Rod Max Count"(u32 500 ("y")) -> ()  [unwired: 1 in, 1 out]
        n139 = shared-variable ".\\local SCA shared var lib.lvlib\\Wheel GV Min Count"(70 ("Wheel GV Min Time")) -> ()  [unwired: 1 in, 1 out]
        n140 = shared-variable ".\\local SCA shared var lib.lvlib\\Sample Rod Min Count"(u32 10 ("y")) -> ()  [unwired: 1 in, 1 out]
        n141 = shared-variable ".\\local SCA shared var lib.lvlib\\Sample Rod Max Count"(u32 1000 ("y")) -> ()  [unwired: 1 in, 1 out]
        n142 = shared-variable ".\\local SCA shared var lib.lvlib\\Retract Rod Max Count"(u32 200 ("y")) -> ()  [unwired: 1 in, 1 out]
        n143 = shared-variable ".\\local SCA shared var lib.lvlib\\Retract Rod Min Count"(u32 30 ("y")) -> ()  [unwired: 1 in, 1 out]
      }
      frame "wait", Default {
        w229 = u32 0
        n144 = shared-variable ".\\local SCA shared var lib.lvlib\\SCA state control"() -> (w225:T5)  [unwired: 1 in, 1 out]
        n145 = case shown="\"change sample\"" w225 {
          tunnel: [w234 w235 w236 w237 w238 w239 w240 w241 w242 w243 w244 w245 w246] -> w227
          frame "wheel GV close" {
            w234 = T5[] [enum."wheel GV close", enum."wait"] items=["initialize", "wait", "change sample start", "change sample", "check position", "wait position", "rotate wheel", "sample change complete", "sample rod up", "sample rod down", "retract rod in", "retract rod out", "insert rod in", "insert rod out", "wheel GV open", "wheel GV close", "vent source", "pump source"]
          }
          frame "wheel GV open" {
            w235 = T5[] [enum."wheel GV open", enum."wait"] items=["initialize", "wait", "change sample start", "change sample", "check position", "wait position", "rotate wheel", "sample change complete", "sample rod up", "sample rod down", "retract rod in", "retract rod out", "insert rod in", "insert rod out", "wheel GV open", "wheel GV close", "vent source", "pump source"]
          }
          frame "sample rod up" {
            w236 = T5[] [enum."sample rod up", enum."wait"] items=["initialize", "wait", "change sample start", "change sample", "check position", "wait position", "rotate wheel", "sample change complete", "sample rod up", "sample rod down", "retract rod in", "retract rod out", "insert rod in", "insert rod out", "wheel GV open", "wheel GV close", "vent source", "pump source"]
          }
          frame "sample rod down" {
            w237 = T5[] [enum."sample rod down", enum."wait"] items=["initialize", "wait", "change sample start", "change sample", "check position", "wait position", "rotate wheel", "sample change complete", "sample rod up", "sample rod down", "retract rod in", "retract rod out", "insert rod in", "insert rod out", "wheel GV open", "wheel GV close", "vent source", "pump source"]
          }
          frame "retract rod in" {
            w238 = T5[] [enum."retract rod in", enum."wait"] items=["initialize", "wait", "change sample start", "change sample", "check position", "wait position", "rotate wheel", "sample change complete", "sample rod up", "sample rod down", "retract rod in", "retract rod out", "insert rod in", "insert rod out", "wheel GV open", "wheel GV close", "vent source", "pump source"]
          }
          frame "retract rod out" {
            w239 = T5[] [enum."retract rod out", enum."wait"] items=["initialize", "wait", "change sample start", "change sample", "check position", "wait position", "rotate wheel", "sample change complete", "sample rod up", "sample rod down", "retract rod in", "retract rod out", "insert rod in", "insert rod out", "wheel GV open", "wheel GV close", "vent source", "pump source"]
          }
          frame "insert rod in" {
            w240 = T5[] [enum."insert rod in", enum."wait"] items=["initialize", "wait", "change sample start", "change sample", "check position", "wait position", "rotate wheel", "sample change complete", "sample rod up", "sample rod down", "retract rod in", "retract rod out", "insert rod in", "insert rod out", "wheel GV open", "wheel GV close", "vent source", "pump source"]
          }
          frame "insert rod out" {
            w241 = T5[] [enum."insert rod out", enum."wait"] items=["initialize", "wait", "change sample start", "change sample", "check position", "wait position", "rotate wheel", "sample change complete", "sample rod up", "sample rod down", "retract rod in", "retract rod out", "insert rod in", "insert rod out", "wheel GV open", "wheel GV close", "vent source", "pump source"]
          }
          frame "rotate wheel" {
            w242 = T5[] [enum."check position", enum."wait"] items=["initialize", "wait", "change sample start", "change sample", "check position", "wait position", "rotate wheel", "sample change complete", "sample rod up", "sample rod down", "retract rod in", "retract rod out", "insert rod in", "insert rod out", "wheel GV open", "wheel GV close", "vent source", "pump source"]
          }
          frame "change sample" {
            w243 = T5[] [enum."change sample start", enum."sample rod up", enum."retract rod in", enum."retract rod out", enum."check position", enum."insert rod in", enum."insert rod out", enum."sample rod down", enum."sample change complete", enum."wait"] items=["initialize", "wait", "change sample start", "change sample", "check position", "wait position", "rotate wheel", "sample change complete", "sample rod up", "sample rod down", "retract rod in", "retract rod out", "insert rod in", "insert rod out", "wheel GV open", "wheel GV close", "vent source", "pump source"]
          }
          frame "vent source" {
            w244 = T5[] [enum."sample rod up", enum."retract rod in", enum."retract rod out", enum."insert rod out", enum."wheel GV close", enum."wait"] items=["initialize", "wait", "change sample start", "change sample", "check position", "wait position", "rotate wheel", "sample change complete", "sample rod up", "sample rod down", "retract rod in", "retract rod out", "insert rod in", "insert rod out", "wheel GV open", "wheel GV close", "vent source", "pump source"]
          }
          frame "pump source" {
            w245 = T5[] [enum."wheel GV open", enum."sample rod up", enum."check position", enum."insert rod in", enum."insert rod out", enum."sample rod down", enum."wait"] items=["initialize", "wait", "change sample start", "change sample", "check position", "wait position", "rotate wheel", "sample change complete", "sample rod up", "sample rod down", "retract rod in", "retract rod out", "insert rod in", "insert rod out", "wheel GV open", "wheel GV close", "vent source", "pump source"]
          }
          frame "wait", Default {
            w246 = T5[] [enum."wait"] items=["initialize", "wait", "change sample start", "change sample", "check position", "wait position", "rotate wheel", "sample change complete", "sample rod up", "sample rod down", "retract rod in", "retract rod out", "insert rod in", "insert rod out", "wheel GV open", "wheel GV close", "vent source", "pump source"]
          }
        }
        n146 = Select(t="Ready", s="clear error", f=w232) -> (s? t:f=w231:string)
        n147 = Index Array(array=w227, index=0) -> (element=w226:T5)
      }
      frame "change sample start" {
        w251 = u32 0
        n148 = Index Array(array=w248, index=1) -> (element=w256:T5)
        n149 = shared-variable "SCA-cRIO\\shared var lib.lvlib\\change sample start end"(FALSE ("change sample start end")) -> ()  [unwired: 1 in, 1 out]
        n150 = shared-variable ".\\local SCA shared var lib.lvlib\\Changing Sample"(TRUE ("Changing Sample")) -> ()  [unwired: 1 in, 1 out]
        n151 = Select(t="Ready", s="clear error 2", f=w254) -> (s? t:f=w253:string)
      }
      frame "sample change complete" {
        w261 = u32 0
        n152 = shared-variable "SCA-cRIO\\shared var lib.lvlib\\change sample start end"(TRUE ("change sample start end")) -> ()  [unwired: 1 in, 1 out]
        n153 = shared-variable ".\\local SCA shared var lib.lvlib\\Changing Sample"(FALSE ("Changing Sample")) -> ()  [unwired: 1 in, 1 out]
        n154 = Array Size(array=w258) -> (size(s)=w259:i32)
        n155 = Index Array(array=w258, index=w259) -> (element=w266:T5)
        n156 = Select(t="Ready", s="clear error 3", f=w264) -> (s? t:f=w263:string)
      }
      frame "wheel GV open" {
        n157 = call "Modify array of SCA states.vi"("Current State"=w275, "Array of states to process"=w276) -> ("Next State"=w277:T5)  [unwired: 7 in, 1 out]
        n158 = shared-variable "SCA-cRIO\\Mod8\\Wheel GV Actuator"(TRUE ("sc gate valve")) -> (error out=w273:errorcluster)  [unwired: 1 in]
        n159 = shared-variable "SCA-cRIO\\global SCA shared var lib.lvlib\\Wheel GV Status"(error in=w273) -> (w272:enum16{"status unclear", "closed", "open"})  [unwired: 1 out]
        n160 = shared-variable ".\\local SCA shared var lib.lvlib\\Wheel GV Min Count"() -> (w267:i32)  [unwired: 1 in, 1 out]
        n161 = Equal?(x=enum16{"status unclear", "closed", "open"}."open", y=w272) -> (x = y?=w270:bool)
        n162 = Select(t=w283, s=w270, f=u32 0) -> (s? t:f=w286:u32)
        n163 = Increment(x=w286) -> (x+1=w282:u32)
        n164 = Greater Or Equal?(x=w282, y=w267) -> (x >= y?=w284:bool)
        n165 = Select(t=w277, s=w284, f=w275) -> (s? t:f=w280:T5)
        n166 = Increment(x=w281) -> (x+1=w268:u32)
        n167 = Format Into String(format string="%s", w275) -> (resulting string=w279:string)  [unwired: 2 in, 1 out]
      }
      frame "wheel GV close" {
        n168 = call "Modify array of SCA states.vi"("Current State"=w293, "Array of states to process"=w294) -> ("Next State"=w295:T5)  [unwired: 7 in, 1 out]
        n169 = shared-variable "SCA-cRIO\\Mod8\\Wheel GV Actuator"(FALSE ("sc gate valve")) -> (error out=w291:errorcluster)  [unwired: 1 in]
        n170 = shared-variable "SCA-cRIO\\global SCA shared var lib.lvlib\\Wheel GV Status"(error in=w291) -> (w290:enum16{"status unclear", "closed", "open"})  [unwired: 1 out]
        n171 = shared-variable ".\\local SCA shared var lib.lvlib\\Wheel GV Min Count"() -> (w306:i32)  [unwired: 1 in, 1 out]
        n172 = Equal?(x=enum16{"status unclear", "closed", "open"}."closed", y=w290) -> (x = y?=w288:bool)
        n173 = Select(t=w302, s=w288, f=u32 0) -> (s? t:f=w305:u32)
        n174 = Increment(x=w305) -> (x+1=w301:u32)
        n175 = Greater Or Equal?(x=w301, y=w306) -> (x >= y?=w303:bool)
        n176 = Select(t=w295, s=w303, f=w293) -> (s? t:f=w299:T5)
        n177 = Increment(x=w300) -> (x+1=w297:u32)
        n178 = Format Into String(format string="%s", w293) -> (resulting string=w298:string)  [unwired: 2 in, 1 out]
      }
      frame "sample rod up" {
        n179 = Increment(x=w323) -> (x+1=w309:u32)
        n180 = shared-variable "SCA-cRIO\\Mod8\\Sample Rod Actuator"(FALSE ("Sample Rod Actuator")) -> (error out=w314:errorcluster)  [unwired: 1 in]
        n181 = shared-variable ".\\local SCA shared var lib.lvlib\\Sample Rod Max Count"() -> (w308:u32)  [unwired: 1 in, 1 out]
        n182 = call "Modify array of SCA states.vi"("Current State"=w316, "Array of states to process"=w317) -> ("Next State"=w318:T5)  [unwired: 7 in, 1 out]
        n183 = shared-variable "SCA-cRIO\\global SCA shared var lib.lvlib\\Sample Rod status"(error in=w314) -> (w313:T3)  [unwired: 1 out]
        n184 = Greater Or Equal?(x=w309, y=w308) -> (x >= y?=w322:bool)
        n185 = shared-variable ".\\local SCA shared var lib.lvlib\\Sample Rod Min Count"() -> (w307:u32)  [unwired: 1 in, 1 out]
        n186 = Equal?(x=w313, y=Vertical_Rod_states."rod up") -> (x = y?=w311:bool)
        n187 = Select(t=w330, s=w311, f=u32 0) -> (s? t:f=w328:u32)
        n188 = Increment(x=w328) -> (x+1=w310:u32)
        n189 = Greater Or Equal?(x=w310, y=w307) -> (x >= y?=w329:bool)
        n190 = Select(t=w318, s=w329, f=w316) -> (s? t:f=w325:T5)
        n191 = case shown="True" w322 {
          tunnel: [w336 u32 0] -> w321
          tunnel: [w334 w337] -> w319
          tunnel: [w335 SCA_states."wait" ("SC2 state")] -> w324
          tunnel: w309 -> [w336 _]
          tunnel: w316 -> [w332 _]
          tunnel: [w331 "sample rod failure"] -> w326
          tunnel: w325 -> [w335 _]
          tunnel: w317 -> [w334 _]
          frame False {
            n192 = Format Into String(format string="%s", w332) -> (resulting string=w331:string)  [unwired: 2 in, 1 out]
          }
          frame True {
            w337 = T5[] [enum."wait", enum."insert rod out", enum."wait"] items=["initialize", "wait", "change sample start", "change sample", "check position", "wait position", "rotate wheel", "sample change complete", "sample rod up", "sample rod down", "retract rod in", "retract rod out", "insert rod in", "insert rod out", "wheel GV open", "wheel GV close", "vent source", "pump source"]
          }
        }
      }
      frame "sample rod down" {
        n193 = Increment(x=w357) -> (x+1=w343:u32)
        n194 = shared-variable "SCA-cRIO\\Mod8\\Sample Rod Actuator"(TRUE ("Sample Rod Actuator")) -> (error out=w348:errorcluster)  [unwired: 1 in]
        n195 = shared-variable ".\\local SCA shared var lib.lvlib\\Sample Rod Max Count"() -> (w341:u32)  [unwired: 1 in, 1 out]
        n196 = call "Modify array of SCA states.vi"("Current State"=w350, "Array of states to process"=w351) -> ("Next State"=w352:T5)  [unwired: 7 in, 1 out]
        n197 = shared-variable "SCA-cRIO\\global SCA shared var lib.lvlib\\Sample Rod status"(error in=w348) -> (w347:T3)  [unwired: 1 out]
        n198 = Greater Or Equal?(x=w343, y=w341) -> (x >= y?=w356:bool)
        n199 = shared-variable ".\\local SCA shared var lib.lvlib\\Sample Rod Min Count"() -> (w342:u32)  [unwired: 1 in, 1 out]
        n200 = Equal?(x=w347, y=Vertical_Rod_states."rod down") -> (x = y?=w345:bool)
        n201 = Select(t=w364, s=w345, f=u32 0) -> (s? t:f=w362:u32)
        n202 = Increment(x=w362) -> (x+1=w344:u32)
        n203 = Greater Or Equal?(x=w344, y=w342) -> (x >= y?=w363:bool)
        n204 = Select(t=w352, s=w363, f=w350) -> (s? t:f=w359:T5)
        n205 = case shown="True" w356 {
          tunnel: [w370 u32 0] -> w355
          tunnel: [w368 w371] -> w353
          tunnel: [w369 SCA_states."wait" ("SC2 state")] -> w358
          tunnel: w343 -> [w370 _]
          tunnel: w350 -> [w366 _]
          tunnel: [w365 "sample rod failure"] -> w360
          tunnel: w359 -> [w369 _]
          tunnel: w351 -> [w368 _]
          frame False {
            n206 = Format Into String(format string="%s", w366) -> (resulting string=w365:string)  [unwired: 2 in, 1 out]
          }
          frame True {
            w371 = T5[] [enum."wait", enum."insert rod out", enum."wait"] items=["initialize", "wait", "change sample start", "change sample", "check position", "wait position", "rotate wheel", "sample change complete", "sample rod up", "sample rod down", "retract rod in", "retract rod out", "insert rod in", "insert rod out", "wheel GV open", "wheel GV close", "vent source", "pump source"]
          }
        }
      }
      frame "retract rod in" {
        n207 = Increment(x=w391) -> (x+1=w378:u32)
        n208 = shared-variable "SCA-cRIO\\Mod8\\Retract Rod Actuator"(TRUE ("Sample Rod Actuator")) -> (error out=w382:errorcluster)  [unwired: 1 in]
        n209 = shared-variable ".\\local SCA shared var lib.lvlib\\Retract Rod Max Count"() -> (w376:u32)  [unwired: 1 in, 1 out]
        n210 = call "Modify array of SCA states.vi"("Current State"=w384, "Array of states to process"=w385) -> ("Next State"=w386:T5)  [unwired: 7 in, 1 out]
        n211 = shared-variable "SCA-cRIO\\global SCA shared var lib.lvlib\\Retract Rod Status"(error in=w382) -> (w381:T2)  [unwired: 1 out]
        n212 = Greater Or Equal?(x=w378, y=w376) -> (x >= y?=w390:bool)
        n213 = shared-variable ".\\local SCA shared var lib.lvlib\\Retract Rod Min Count"() -> (w375:u32)  [unwired: 1 in, 1 out]
        n214 = Equal?(x=w381, y=Horizontal_Rod_states."rod in" ("Enum")) -> (x = y?=w380:bool)
        n215 = Select(t=w398, s=w380, f=u32 0) -> (s? t:f=w396:u32)
        n216 = Increment(x=w396) -> (x+1=w379:u32)
        n217 = Greater Or Equal?(x=w379, y=w375) -> (x >= y?=w397:bool)
        n218 = Select(t=w386, s=w397, f=w384) -> (s? t:f=w393:T5)
        n219 = case shown="True" w390 {
          tunnel: [w404 u32 0] -> w389
          tunnel: [w402 w405] -> w387
          tunnel: [w403 SCA_states."retract rod out" ("SC2 state")] -> w392
          tunnel: w378 -> [w404 _]
          tunnel: w384 -> [w400 _]
          tunnel: [w399 "retract rod failure"] -> w394
          tunnel: w393 -> [w403 _]
          tunnel: w385 -> [w402 _]
          frame False {
            n220 = Format Into String(format string="%s", w400) -> (resulting string=w399:string)  [unwired: 2 in, 1 out]
          }
          frame True {
            w405 = T5[] [enum."retract rod out", enum."insert rod out", enum."wait"] items=["initialize", "wait", "change sample start", "change sample", "check position", "wait position", "rotate wheel", "sample change complete", "sample rod up", "sample rod down", "retract rod in", "retract rod out", "insert rod in", "insert rod out", "wheel GV open", "wheel GV close", "vent source", "pump source"]
          }
        }
      }
      frame "retract rod out" {
        n221 = Increment(x=w425) -> (x+1=w412:u32)
        n222 = shared-variable "SCA-cRIO\\Mod8\\Retract Rod Actuator"(FALSE ("Sample Rod Actuator")) -> (error out=w416:errorcluster)  [unwired: 1 in]
        n223 = call "Modify array of SCA states.vi"("Current State"=w418, "Array of states to process"=w419) -> ("Next State"=w420:T5)  [unwired: 7 in, 1 out]
        n224 = shared-variable ".\\local SCA shared var lib.lvlib\\Retract Rod Max Count"() -> (w410:u32)  [unwired: 1 in, 1 out]
        n225 = shared-variable "SCA-cRIO\\global SCA shared var lib.lvlib\\Retract Rod Status"(error in=w416) -> (w415:T2)  [unwired: 1 out]
        n226 = Greater Or Equal?(x=w412, y=w410) -> (x >= y?=w424:bool)
        n227 = shared-variable ".\\local SCA shared var lib.lvlib\\Retract Rod Min Count"() -> (w409:u32)  [unwired: 1 in, 1 out]
        n228 = Equal?(x=w415, y=Horizontal_Rod_states."rod out" ("Enum")) -> (x = y?=w414:bool)
        n229 = Select(t=w432, s=w414, f=u32 0) -> (s? t:f=w430:u32)
        n230 = Increment(x=w430) -> (x+1=w413:u32)
        n231 = Greater Or Equal?(x=w413, y=w409) -> (x >= y?=w431:bool)
        n232 = Select(t=w420, s=w431, f=w418) -> (s? t:f=w427:T5)
        n233 = case shown="True" w424 {
          tunnel: [w438 u32 0] -> w423
          tunnel: [w436 w439] -> w421
          tunnel: [w437 SCA_states."retract rod out" ("SC2 state")] -> w426
          tunnel: w412 -> [w438 _]
          tunnel: w418 -> [w434 _]
          tunnel: [w433 "retract rod failure"] -> w428
          tunnel: w427 -> [w437 _]
          tunnel: w419 -> [w436 _]
          frame False {
            n234 = Format Into String(format string="%s", w434) -> (resulting string=w433:string)  [unwired: 2 in, 1 out]
          }
          frame True {
            w439 = T5[] [enum."retract rod out", enum."insert rod out", enum."wait"] items=["initialize", "wait", "change sample start", "change sample", "check position", "wait position", "rotate wheel", "sample change complete", "sample rod up", "sample rod down", "retract rod in", "retract rod out", "insert rod in", "insert rod out", "wheel GV open", "wheel GV close", "vent source", "pump source"]
          }
        }
      }
      frame "insert rod in" {
        n235 = Increment(x=w459) -> (x+1=w446:u32)
        n236 = shared-variable "SCA-cRIO\\Mod8\\Insert Rod Actuator"(TRUE ("Sample Rod Actuator")) -> (error out=w450:errorcluster)  [unwired: 1 in]
        n237 = call "Modify array of SCA states.vi"("Current State"=w452, "Array of states to process"=w453) -> ("Next State"=w454:T5)  [unwired: 7 in, 1 out]
        n238 = shared-variable ".\\local SCA shared var lib.lvlib\\Insert Rod Max Count"() -> (w444:u32)  [unwired: 1 in, 1 out]
        n239 = shared-variable "SCA-cRIO\\global SCA shared var lib.lvlib\\Insert Rod Status"(error in=w450) -> (w449:T2)  [unwired: 1 out]
        n240 = Greater Or Equal?(x=w446, y=w444) -> (x >= y?=w458:bool)
        n241 = shared-variable ".\\local SCA shared var lib.lvlib\\Insert Rod Min Count"() -> (w443:u32)  [unwired: 1 in, 1 out]
        n242 = Equal?(x=w449, y=Horizontal_Rod_states."rod in" ("Enum")) -> (x = y?=w448:bool)
        n243 = Select(t=w466, s=w448, f=u32 0) -> (s? t:f=w464:u32)
        n244 = Increment(x=w464) -> (x+1=w447:u32)
        n245 = Greater Or Equal?(x=w447, y=w443) -> (x >= y?=w465:bool)
        n246 = Select(t=w454, s=w465, f=w452) -> (s? t:f=w461:T5)
        n247 = case shown="True" w458 {
          tunnel: [w472 u32 0] -> w457
          tunnel: [w470 w473] -> w455
          tunnel: [w471 SCA_states."insert rod out" ("SC2 state")] -> w460
          tunnel: w446 -> [w472 _]
          tunnel: w452 -> [w468 _]
          tunnel: [w467 "insert rod failure"] -> w462
          tunnel: w461 -> [w471 _]
          tunnel: w453 -> [w470 _]
          frame False {
            n248 = Format Into String(format string="%s", w468) -> (resulting string=w467:string)  [unwired: 2 in, 1 out]
          }
          frame True {
            w473 = T5[] [enum."insert rod out", enum."retract rod out", enum."wait"] items=["initialize", "wait", "change sample start", "change sample", "check position", "wait position", "rotate wheel", "sample change complete", "sample rod up", "sample rod down", "retract rod in", "retract rod out", "insert rod in", "insert rod out", "wheel GV open", "wheel GV close", "vent source", "pump source"]
          }
        }
      }
      frame "insert rod out" {
        n249 = Increment(x=w493) -> (x+1=w480:u32)
        n250 = shared-variable ".\\local SCA shared var lib.lvlib\\Insert Rod Max Count"() -> (w478:u32)  [unwired: 1 in, 1 out]
        n251 = shared-variable "SCA-cRIO\\Mod8\\Insert Rod Actuator"(FALSE ("Sample Rod Actuator")) -> (error out=w484:errorcluster)  [unwired: 1 in]
        n252 = call "Modify array of SCA states.vi"("Current State"=w486, "Array of states to process"=w487) -> ("Next State"=w488:T5)  [unwired: 7 in, 1 out]
        n253 = shared-variable "SCA-cRIO\\global SCA shared var lib.lvlib\\Insert Rod Status"(error in=w484) -> (w483:T2)  [unwired: 1 out]
        n254 = Greater Or Equal?(x=w480, y=w478) -> (x >= y?=w492:bool)
        n255 = shared-variable ".\\local SCA shared var lib.lvlib\\Insert Rod Min Count"() -> (w477:u32)  [unwired: 1 in, 1 out]
        n256 = Equal?(x=w483, y=Horizontal_Rod_states."rod out" ("Enum")) -> (x = y?=w482:bool)
        n257 = Select(t=w500, s=w482, f=u32 0) -> (s? t:f=w498:u32)
        n258 = Increment(x=w498) -> (x+1=w481:u32)
        n259 = Greater Or Equal?(x=w481, y=w477) -> (x >= y?=w499:bool)
        n260 = Select(t=w488, s=w499, f=w486) -> (s? t:f=w495:T5)
        n261 = case shown="True" w492 {
          tunnel: [w506 u32 0] -> w491
          tunnel: [w504 w507] -> w489
          tunnel: [w505 SCA_states."insert rod out" ("SC2 state")] -> w494
          tunnel: w480 -> [w506 _]
          tunnel: w486 -> [w502 _]
          tunnel: [w501 "insert rod failure"] -> w496
          tunnel: w495 -> [w505 _]
          tunnel: w487 -> [w504 _]
          frame False {
            n262 = Format Into String(format string="%s", w502) -> (resulting string=w501:string)  [unwired: 2 in, 1 out]
          }
          frame True {
            w507 = T5[] [enum."insert rod out", enum."retract rod out", enum."wait"] items=["initialize", "wait", "change sample start", "change sample", "check position", "wait position", "rotate wheel", "sample change complete", "sample rod up", "sample rod down", "retract rod in", "retract rod out", "insert rod in", "insert rod out", "wheel GV open", "wheel GV close", "vent source", "pump source"]
          }
        }
      }
      frame "rotate wheel" {
        w536 = 10000.0 ("acceleration")
        # "in motor steps"
        n263 = shared-variable "SCA-cRIO\\global SCA shared var lib.lvlib\\New Move"() -> (w519:dbl)  [unwired: 1 in, 1 out]
        n264 = Increment(x=w533) -> (x+1=w528:u32)
        n265 = Increment(x=w535) -> (x+1=w518:u32)
        n266 = shared-variable ".\\local SCA shared var lib.lvlib\\Motor Status"(FALSE ("Motor Status")) -> ()  [unwired: 1 in, 1 out]
        n267 = feedback #1() -> (w513:bool)  [unwired: 1 in]
        n268 = xnode "Straight-Line Move"("resource"=w537, "execute"=w513, "position"=w519, "velocity"=w536, "acceleration"=w536, "deceleration"=w536, "accel. jerk"=w536, "smoothing"=w536) -> ("error out"=w516:errorcluster, "done"=w524:bool)  [unwired: 2 in, 4 out]
        "done" <- w524
        "Rotate Wheel error" <- w516
        n269 = shared-variable ".\\local SCA shared var lib.lvlib\\Rotate Wheel Min Count"() -> (w512:u32)  [unwired: 1 in, 1 out]
        n270 = shared-variable ".\\local SCA shared var lib.lvlib\\Rotate Wheel error"(w516) -> ()  [unwired: 1 in, 1 out]
        n271 = Not(x=w524) -> (.not. x?=w514:bool)
        n272 = feedback-in #1(w514) -> ()
        n273 = local write "Execute Move"(w514) -> ()
        n274 = shared-variable ".\\local SCA shared var lib.lvlib\\Rotate Wheel Max Count"() -> (w511:u32)  [unwired: 1 in, 1 out]
        n275 = Greater Or Equal?(x=w518, y=w512) -> (x >= y?=w529:bool)
        n276 = Select(t=u32 0, s=w529, f=w528) -> (s? t:f=w526:u32)
        n277 = Select(t=SCA_states."wait position" ("SC2 state"), s=w524, f=SCA_states."rotate wheel" ("SC2 state")) -> (s? t:f=w525:T5)
        n278 = Greater Or Equal?(x=w528, y=w511) -> (x >= y?=w534:bool)
        n279 = case shown="False" w534 {
          tunnel: [w538 w543] -> w532
          tunnel: [w542 SCA_states."retract rod out" ("SC2 state")] -> w531
          tunnel: w522 -> [w540 _]
          tunnel: [w539 "rotate failure"] -> w530
          tunnel: w525 -> [w542 _]
          tunnel: w523 -> [w538 _]
          frame False {
            n280 = Format Into String(format string="%s", w540) -> (resulting string=w539:string)  [unwired: 2 in, 1 out]
          }
          frame True {
            w543 = T5[] [enum."retract rod out", enum."insert rod out", enum."wait"] items=["initialize", "wait", "change sample start", "change sample", "check position", "wait position", "rotate wheel", "sample change complete", "sample rod up", "sample rod down", "retract rod in", "retract rod out", "insert rod in", "insert rod out", "wheel GV open", "wheel GV close", "vent source", "pump source"]
          }
        }
      }
      frame "wait position" {
        n281 = Increment(x=w588) -> (x+1=w589:u32)
        n282 = Increment(x=w586) -> (x+1=w582:u32)
        n283 = Greater Or Equal?(x=w589, y=u32 8000) -> (x >= y?=w583:bool)
        n284 = Select(t=u32 0, s=w583, f=w582) -> (s? t:f=w580:u32)
        n285 = Greater Or Equal?(x=w582, y=u32 1500) -> (x >= y?=w579:bool)
        n286 = case shown="False" w579 {
          tunnel: [w593 w594] -> w585
          tunnel: w576 -> [w591 _]
          tunnel: [w590 "rotate failure"] -> w584
          tunnel: w575 -> [w593 _]
          frame False {
            n287 = Format Into String(format string="%s", w591) -> (resulting string=w590:string)  [unwired: 2 in, 1 out]
          }
          frame True {
            w594 = T5[] [enum."retract rod out", enum."insert rod out", enum."wait"] items=["initialize", "wait", "change sample start", "change sample", "check position", "wait position", "rotate wheel", "sample change complete", "sample rod up", "sample rod down", "retract rod in", "retract rod out", "insert rod in", "insert rod out", "wheel GV open", "wheel GV close", "vent source", "pump source"]
          }
        }
        n288 = Select(t=SCA_states."wait position" ("SC2 state"), s=w579, f=SCA_states."check position" ("SC2 state")) -> (s? t:f=w578:T5)
      }
      frame "check position" {
        # "Move in motor steps"
        n289 = shared-variable "SCA-cRIO\\global SCA shared var lib.lvlib\\Encoder position"() -> (w601:i16)  [unwired: 1 in, 1 out]
        n290 = shared-variable "SCA-cRIO\\global SCA shared var lib.lvlib\\Encoder Offset"() -> (w602:i16)  [unwired: 1 in, 1 out]
        n291 = shared-variable ".\\local SCA shared var lib.lvlib\\New sample"() -> (w598:i8)  [unwired: 1 in, 1 out]
        n292 = call "SCA Sample-Encoder conversion.vi"("Step Window Radius"="Step Window Radius", "Rollover Sample"="Rollover Sample", "Encoder Offset"=w601, "Encoder Position"=w602, "Desired Sample"=w598) -> ("Window limit 1"=w597:i16, "Within Range?"=w610:bool, "Encoder destination"=w608:i16, "Window limit 2"=w596:i16, "New move (encoder steps)"=w613:i16)  [unwired: 2 in]
        "Encoder Destination" <- w608
        "In Range?" <- w610
        "Window Limit 2" <- w596
        "Window Limit 1" <- w597
        n293 = shared-variable "SCA-cRIO\\shared var lib.lvlib\\wheel offset plus"(w597) -> ()  [unwired: 1 in, 1 out]
        n294 = shared-variable "SCA-cRIO\\global SCA shared var lib.lvlib\\Encoder Destination"(w608) -> ()  [unwired: 1 in, 1 out]
        n295 = shared-variable "SCA-cRIO\\shared var lib.lvlib\\wheel offset minus"(w596) -> ()  [unwired: 1 in, 1 out]
        n296 = call "Modify array of SCA states.vi"("Current State"=w607, "Array of states to process"=w606) -> ("Next State"=w605:T5)  [unwired: 7 in, 1 out]
        n297 = Select(t=w605, s=w610, f=SCA_states."rotate wheel" ("SC2 state")) -> (s? t:f=w617:T5)
        n298 = shared-variable ".\\local SCA shared var lib.lvlib\\Motor Status"(w610) -> ()  [unwired: 1 in, 1 out]
        n299 = Multiply(x=w613, y=3.0519) -> (x*y=w609:dbl)
        "New Move" <- w609
        n300 = shared-variable "SCA-cRIO\\global SCA shared var lib.lvlib\\New Move"(w609) -> ()  [unwired: 1 in, 1 out]
        n301 = Format Into String(format string="%s", w607) -> (resulting string=w616:string)  [unwired: 2 in, 1 out]
      }
    }
    "action" <- w198
    "SCA next state" <- w202
    n302 = shared-variable "SCA-cRIO\\global SCA shared var lib.lvlib\\Current State"(w192) -> ()  [unwired: 1 in, 1 out]
    n303 = call "Wait Until Next Multiple"("Count(mSec)"=u32 5) -> ()  [unwired: 1 out]
    n304 = shared-variable "SCA-cRIO\\global SCA shared var lib.lvlib\\SC SM counter"(w194) -> ()  [unwired: 1 in, 1 out]
  }
  n305 = while {
    tunnel: w9 -> [w623]
    stop <- FALSE ("stop 3") stop-if-true
    # "Convectron readback - GP375 Convectron uses thermocouple gauge to measure pressure on wheel chamber"
    n306 = Concatenate Strings("RD" ("write buffer 2"), "\r") -> (w630:string)
    n307 = Wait Until Next ms Multiple(millisecond multiple=u32 2000) -> ()  [unwired: 1 out]
    n308 = VISA Write(VISA resource name=w623, write buffer=w630) -> (VISA resource name out=w624:refnum<visa-resource-name>, error out=w620:errorcluster)  [unwired: 1 in, 1 out]
    n309 = property class="Instr"(reference=w624, error in=w620) -> (reference out=w625:refnum<visa-resource-name>, error out=w619:errorcluster, "Bytes at Port"=w626:u32)
    n310 = VISA Read(VISA resource name=w625, byte count=w626, error in (no error)=w619) -> (read buffer=w621:string, error out=w618:errorcluster)  [unwired: 2 out]
    "Sample Wheel Convectron" <- w621
    "Convectron readback loop error" <- w618
    n311 = shared-variable ".\\local SCA shared var lib.lvlib\\Convectron readback loop error"(w618) -> ()  [unwired: 1 in, 1 out]
    n312 = shared-variable "SCA-cRIO\\global SCA shared var lib.lvlib\\Sample Wheel Convectron"(w621) -> ()  [unwired: 1 in, 1 out]
  }
  n313 = while {
    tunnel: w14 -> [w634]
    tunnel: w20 -> [w637]
    stop <- FALSE ("stop 4") stop-if-true
    w633 = 3.0 ("Delay Time (s)")
    # "GP307 readback for both controllers on SCA - Bellows readings in and around sample rods upper position; Ion source readings are in and around source region"
    n314 = Wait Until Next ms Multiple(millisecond multiple=u32 500) -> ()  [unwired: 1 out]
    n315 = call "GP307 Read-RT.vi"("Delay Time (s)"=w633, "VISA Refnum in"=w637) -> ("error out"=w635:errorcluster, "GP307 output"=w636:T1)  [unwired: 7 in, 1 out]
    "Bellows Vac Cluster" <- w636
    n316 = call "GP307 Read-RT.vi"("Delay Time (s)"=w633, "VISA Refnum in"=w634) -> ("error out"=w631:errorcluster, "GP307 output"=w632:T1)  [unwired: 7 in, 1 out]
    "Ion Source Vac Cluster" <- w632
    n317 = shared-variable "SCA-cRIO\\global SCA shared var lib.lvlib\\Bellows Vac Cluster"(w636) -> ()  [unwired: 1 in, 1 out]
    n318 = shared-variable "SCA-cRIO\\global SCA shared var lib.lvlib\\Ion Source Vac Cluster"(w632) -> ()  [unwired: 1 in, 1 out]
    n319 = Merge Errors(w635, w631) -> (w638:errorcluster)
    "Vac Readback Loop error" <- w638
    n320 = shared-variable ".\\local SCA shared var lib.lvlib\\Vac Readback Loop error"(w638) -> ()  [unwired: 1 in, 1 out]
  }
  n321 = while {
    stop <- FALSE stop-if-true
    n322 = shared-variable "SCA-cRIO\\global SCA shared var lib.lvlib\\Pump out Source"() -> (w642:bool)  [unwired: 1 in, 1 out]
    "Pumping out Source" <- w642
    n323 = Wait Until Next ms Multiple(millisecond multiple=u32 100) -> ()  [unwired: 1 out]
    n324 = case shown="True" w642 {
      frame False {
      }
      frame True {
        n325 = shared-variable "SCA-cRIO\\global SCA shared var lib.lvlib\\Pump out Source"(FALSE ("rod up shared")) -> ()  [unwired: 1 in, 1 out]
        n326 = shared-variable ".\\local SCA shared var lib.lvlib\\SCA state control"(SCA_states."pump source" ("SC2 state")) -> ()  [unwired: 1 in, 1 out]
      }
    }
  }
  n327 = while {
    stop <- FALSE stop-if-true
    n328 = shared-variable "SCA-cRIO\\global SCA shared var lib.lvlib\\Close Wheel GV"() -> (w646:bool)  [unwired: 1 in, 1 out]
    "Close Wheel GV" <- w646
    n329 = Wait Until Next ms Multiple(millisecond multiple=u32 50) -> ()  [unwired: 1 out]
    n330 = case shown="True" w646 {
      frame False {
      }
      frame True {
        n331 = shared-variable "SCA-cRIO\\global SCA shared var lib.lvlib\\Close Wheel GV"(FALSE ("rod up shared")) -> ()  [unwired: 1 in, 1 out]
        n332 = shared-variable ".\\local SCA shared var lib.lvlib\\SCA state control"(SCA_states."wheel GV close" ("SC2 state")) -> ()  [unwired: 1 in, 1 out]
      }
    }
  }
  n333 = while {
    stop <- FALSE ("stop") stop-if-true
    n334 = shared-variable "SCA-cRIO\\Mod7\\Wheel GV OPEN sensor"() -> (w674:bool, error out=w660:errorcluster)  [unwired: 1 in]
    n335 = shared-variable "SCA-cRIO\\Mod7\\Wheel GV CLOSED sensor"(error in=w660) -> (w675:bool, error out=w659:errorcluster)
    n336 = Wait Until Next ms Multiple(millisecond multiple=u32 50) -> ()  [unwired: 1 out]
    n337 = shared-variable "SCA-cRIO\\Mod7\\Retract Rod IN sensor"() -> (w669:bool, error out=w662:errorcluster)  [unwired: 1 in]
    "Retract Rod IN sensor" <- w669
    n338 = shared-variable "SCA-cRIO\\Mod7\\Retract Rod OUT sensor"(error in=w662) -> (w668:bool, error out=w656:errorcluster)
    "Retract Rod OUT sensor" <- w668
    n339 = shared-variable "SCA-cRIO\\Mod7\\Insert Rod IN sensor"() -> (w667:bool, error out=w661:errorcluster)  [unwired: 1 in]
    "Insert Rod IN sensor" <- w667
    n340 = shared-variable "SCA-cRIO\\Mod7\\Insert Rod OUT sensor"(error in=w661) -> (w666:bool, error out=w658:errorcluster)
    "Insert Rod OUT sensor" <- w666
    n341 = shared-variable "SCA-cRIO\\Mod7\\Sample Rod UP sensor"() -> (w672:bool, error out=w663:errorcluster)  [unwired: 1 in]
    "Sample Rod UP sensor" <- w672
    n342 = shared-variable "SCA-cRIO\\Mod7\\Sample Rod DOWN sensor"(error in=w663) -> (w671:bool, error out=w657:errorcluster)
    "Sample Rod DOWN sensor" <- w671
    n343 = Bundle By Name(cluster=T4 {"OPEN sensor"=FALSE, "Closed sensor"=FALSE} ("Gate Valve"), "OPEN sensor"=w674, "Closed sensor"=w675) -> (w677:T4)
    "Wheel GV" <- w677
    n344 = call "Horizontal Rod Sensor-State converter.vi"("IN Sensor"=w667, "OUT Sensor"=w666) -> ("Status"=w665:T2)  [unwired: 8 in]
    "Insert Rod Status" <- w665
    n345 = call "Horizontal Rod Sensor-State converter.vi"("IN Sensor"=w669, "OUT Sensor"=w668) -> ("Status"=w664:T2)  [unwired: 8 in]
    "Retract Rod Status" <- w664
    n346 = call "Vertical Rod Sensor-State converter.vi"("UP Sensor"=w672, "DOWN Sensor"=w671) -> ("Status"=w670:T3)  [unwired: 8 in]
    "Sample Rod status" <- w670
    n347 = shared-variable "SCA-cRIO\\global SCA shared var lib.lvlib\\Retract Rod Status"(w664, error in=w656) -> (error out=w653:errorcluster)
    n348 = shared-variable "SCA-cRIO\\global SCA shared var lib.lvlib\\Insert Rod Status"(w665, error in=w658) -> (error out=w652:errorcluster)
    n349 = call "GV status converter.vi"("Gate Valve"=w677) -> ("GV Status"=w673:T6)  [unwired: 10 in]
    n350 = shared-variable "SCA-cRIO\\global SCA shared var lib.lvlib\\Sample Rod status"(w670, error in=w657) -> (error out=w654:errorcluster)
    n351 = shared-variable "SCA-cRIO\\global SCA shared var lib.lvlib\\Wheel GV Status"(w673, error in=w659) -> (error out=w651:errorcluster)
    n352 = Merge Errors(w654, w653, w652, w651) -> (w655:errorcluster)
    "Sensor loop error" <- w655
    n353 = shared-variable ".\\local SCA shared var lib.lvlib\\Sensor Loop error"(w655) -> ()  [unwired: 1 in, 1 out]
  }
  n354 = node-c288() -> (w5:T7)  [unwired: 4 in]
  n355 = timed-loop {
    timing: w5 -> [_]
    timing-out: [_] -> w4
    stop <- FALSE stop-if-true
    # "Encoder readback loop"
    n356 = node-c288() -> ()  [unwired: 1 in, 1 out]
    n357 = shared-variable "SCA-cRIO\\Mod6\\DIO0"() -> (w712:bool, error out=w695:errorcluster)  [unwired: 1 in]
    n358 = shared-variable "SCA-cRIO\\Mod6\\DIO1"(error in=w695) -> (w711:bool, error out=w694:errorcluster)
    n359 = shared-variable "SCA-cRIO\\Mod6\\DIO2"(error in=w694) -> (w702:bool, error out=w693:errorcluster)
    n360 = shared-variable "SCA-cRIO\\Mod6\\DIO3"(error in=w693) -> (w701:bool, error out=w692:errorcluster)
    n361 = shared-variable "SCA-cRIO\\Mod6\\DIO4"(error in=w692) -> (w710:bool, error out=w691:errorcluster)
    n362 = shared-variable "SCA-cRIO\\Mod6\\DIO5"(error in=w691) -> (w709:bool, error out=w690:errorcluster)
    n363 = shared-variable "SCA-cRIO\\Mod6\\DIO6"(error in=w690) -> (w708:bool, error out=w689:errorcluster)
    n364 = shared-variable "SCA-cRIO\\Mod6\\DIO7"(error in=w689) -> (w688:bool, error out=w687:errorcluster)
    n365 = shared-variable "SCA-cRIO\\Mod6\\DIO8"(error in=w687) -> (w707:bool, error out=w686:errorcluster)
    n366 = shared-variable "SCA-cRIO\\Mod6\\DIO9"(error in=w686) -> (w700:bool, error out=w685:errorcluster)
    n367 = shared-variable "SCA-cRIO\\Mod6\\DIO10"(error in=w685) -> (w706:bool, error out=w684:errorcluster)
    n368 = shared-variable "SCA-cRIO\\Mod6\\DIO11"(error in=w684) -> (w705:bool, error out=w683:errorcluster)
    n369 = shared-variable "SCA-cRIO\\Mod6\\DIO12"(error in=w683) -> (w704:bool, error out=w682:errorcluster)
    n370 = shared-variable "SCA-cRIO\\Mod6\\DIO13"(error in=w682) -> (w703:bool, error out=w681:errorcluster)
    n371 = Bundle By Name(cluster=T10 {"MSB"=FALSE, "13th bit"=FALSE, "12th bit"=FALSE, "11th bit"=FALSE, "10th bit"=FALSE, "9th bit"=FALSE, "8th bit"=FALSE, "7th bit"=FALSE, "6th bit"=FALSE, "5th bit"=FALSE, "4th bit"=FALSE, "3rd bit"=FALSE, "2nd bit"=FALSE, "LSB"=FALSE} ("Cluster"), "MSB"=w712, "13th bit"=w711, "12th bit"=w702, "11th bit"=w701, "10th bit"=w710, "9th bit"=w709, "8th bit"=w708, "7th bit"=w688, "6th bit"=w707, "5th bit"=w700, "4th bit"=w706, "3rd bit"=w705, "2nd bit"=w704, "LSB"=w703) -> (w714:T10)
    n372 = call "Encoder-Decoder.vi"("Encoder data"=w714) -> ("Raw bits"=→"Raw bits":bool[], "Converted bits"=→"Converted bits":bool[], "Encoder position"=w699:u16)  [unwired: 8 in]
    "Encoder position" <- w699
    n373 = shared-variable "SCA-cRIO\\global SCA shared var lib.lvlib\\Encoder position"(w699, error in=w681) -> (error out=w680:errorcluster)
    "Encoder loop error" <- w680
    n374 = shared-variable ".\\local SCA shared var lib.lvlib\\Encoder loop error"(w680) -> ()  [unwired: 1 in, 1 out]
    n375 = node-c288() -> ()  [unwired: 1 in, 1 out]
  }
  n376 = while {
    stop <- FALSE stop-if-true
    n377 = shared-variable "SCA-cRIO\\global SCA shared var lib.lvlib\\Sample Rod retraction"() -> (w718:bool)  [unwired: 1 in, 1 out]
    "retract Sample Rod" <- w718
    n378 = Wait Until Next ms Multiple(millisecond multiple=u32 100) -> ()  [unwired: 1 out]
    n379 = case shown="True" w718 {
      frame False {
      }
      frame True {
        n380 = shared-variable "SCA-cRIO\\global SCA shared var lib.lvlib\\Sample Rod retraction"(FALSE ("rod up shared")) -> ()  [unwired: 1 in, 1 out]
        n381 = shared-variable ".\\local SCA shared var lib.lvlib\\SCA state control"(SCA_states."sample rod up" ("SC2 state")) -> ()  [unwired: 1 in, 1 out]
      }
    }
  }
  n382 = while {
    stop <- FALSE stop-if-true
    n383 = shared-variable "SCA-cRIO\\global SCA shared var lib.lvlib\\Insert Rod retraction"() -> (w723:bool)  [unwired: 1 in, 1 out]
    "retract Insert Rod" <- w723
    n384 = Wait Until Next ms Multiple(millisecond multiple=u32 100) -> ()  [unwired: 1 out]
    n385 = case shown="True" w723 {
      frame False {
      }
      frame True {
        n386 = shared-variable "SCA-cRIO\\global SCA shared var lib.lvlib\\Insert Rod retraction"(FALSE ("rod up shared")) -> ()  [unwired: 1 in, 1 out]
        n387 = shared-variable ".\\local SCA shared var lib.lvlib\\SCA state control"(SCA_states."insert rod out" ("SC2 state")) -> ()  [unwired: 1 in, 1 out]
      }
    }
  }
  n388 = while {
    stop <- FALSE stop-if-true
    n389 = shared-variable "SCA-cRIO\\global SCA shared var lib.lvlib\\Retract Rod retraction"() -> (w728:bool)  [unwired: 1 in, 1 out]
    "retract Retract Rod" <- w728
    n390 = Wait Until Next ms Multiple(millisecond multiple=u32 100) -> ()  [unwired: 1 out]
    n391 = case shown="True" w728 {
      frame False {
      }
      frame True {
        n392 = shared-variable "SCA-cRIO\\global SCA shared var lib.lvlib\\Retract Rod retraction"(FALSE ("rod up shared")) -> ()  [unwired: 1 in, 1 out]
        n393 = shared-variable ".\\local SCA shared var lib.lvlib\\SCA state control"(SCA_states."retract rod out" ("SC2 state")) -> ()  [unwired: 1 in, 1 out]
      }
    }
  }
  n394 = while {
    stop <- FALSE stop-if-true
    n395 = shared-variable "SCA-cRIO\\global SCA shared var lib.lvlib\\Retract Rod insertion"() -> (w733:bool)  [unwired: 1 in, 1 out]
    "insert Retract Rod" <- w733
    n396 = Wait Until Next ms Multiple(millisecond multiple=u32 100) -> ()  [unwired: 1 out]
    n397 = case shown="True" w733 {
      frame False {
      }
      frame True {
        n398 = shared-variable "SCA-cRIO\\global SCA shared var lib.lvlib\\Retract Rod insertion"(FALSE ("rod up shared")) -> ()  [unwired: 1 in, 1 out]
        n399 = shared-variable ".\\local SCA shared var lib.lvlib\\SCA state control"(SCA_states."retract rod in" ("SC2 state")) -> ()  [unwired: 1 in, 1 out]
      }
    }
  }
  n400 = while {
    stop <- FALSE stop-if-true
    n401 = shared-variable "SCA-cRIO\\global SCA shared var lib.lvlib\\Sample Rod insertion"() -> (w738:bool)  [unwired: 1 in, 1 out]
    "insert Sample Rod" <- w738
    n402 = Wait Until Next ms Multiple(millisecond multiple=u32 100) -> ()  [unwired: 1 out]
    n403 = case shown="True" w738 {
      frame False {
      }
      frame True {
        n404 = shared-variable "SCA-cRIO\\global SCA shared var lib.lvlib\\Sample Rod insertion"(FALSE ("rod up shared")) -> ()  [unwired: 1 in, 1 out]
        n405 = shared-variable ".\\local SCA shared var lib.lvlib\\SCA state control"(SCA_states."sample rod down" ("SC2 state")) -> ()  [unwired: 1 in, 1 out]
      }
    }
  }
  n406 = while {
    stop <- FALSE stop-if-true
    n407 = shared-variable "SCA-cRIO\\global SCA shared var lib.lvlib\\Insert Rod insertion"() -> (w743:bool)  [unwired: 1 in, 1 out]
    "insert Insert Rod" <- w743
    n408 = Wait Until Next ms Multiple(millisecond multiple=u32 100) -> ()  [unwired: 1 out]
    n409 = case shown="True" w743 {
      frame False {
      }
      frame True {
        n410 = shared-variable "SCA-cRIO\\global SCA shared var lib.lvlib\\Insert Rod insertion"(FALSE ("rod up shared")) -> ()  [unwired: 1 in, 1 out]
        n411 = shared-variable ".\\local SCA shared var lib.lvlib\\SCA state control"(SCA_states."insert rod in" ("SC2 state")) -> ()  [unwired: 1 in, 1 out]
      }
    }
  }
  n412 = node-c288(w4) -> ()  [unwired: 1 out]
  n413 = disable-structure shown="Disabled" {
    frame Disabled {
      n414 = while {
        stop <- FALSE stop-if-true
        # "What is this now?"
        n415 = shared-variable "SCA-cRIO\\shared var lib.lvlib\\rezero"() -> (w748:bool)  [unwired: 1 in, 1 out]
        n416 = Wait Until Next ms Multiple(millisecond multiple=u32 100) -> ()  [unwired: 1 out]
        n417 = case shown="True" w748 {
          frame False {
          }
          frame True {
            n418 = shared-variable "SCA-cRIO\\shared var lib.lvlib\\rezero"(FALSE ("rod up shared")) -> ()  [unwired: 1 in, 1 out]
            n419 = shared-variable ".\\local SCA shared var lib.lvlib\\SCA state control"(SCA_states."initialize" ("SC2 state")) -> ()  [unwired: 1 in, 1 out]
          }
        }
      }
      n420 = local write item#-1(T11 "rezero" ("state control")) -> ()
    }
    frame Enabled {
    }
  }
  n421 = disable-structure shown="Disabled" {
    frame Disabled {
      # "Was in sensor/acutator loop"
      n422 = shared-variable "SCA-cRIO\\shared var lib.lvlib\\change sample start end"() -> (→"change sample start end":bool)  [unwired: 1 in, 1 out]
      n423 = shared-variable "SCA-cRIO\\shared var lib.lvlib\\start sample change"() -> (→"start sample change":bool)  [unwired: 1 in, 1 out]
    }
    frame Enabled {
    }
  }
  n424 = while {
    stop <- FALSE stop-if-true
    # "What is this now?"
    n425 = shared-variable "SCA-cRIO\\shared var lib.lvlib\\set encoder wheel"() -> (w755:bool)  [unwired: 1 in, 1 out]
    n426 = Wait Until Next ms Multiple(millisecond multiple=u32 100) -> ()  [unwired: 1 out]
    n427 = case shown="True" w755 {
      frame False {
      }
      frame True {
        n428 = shared-variable "SCA-cRIO\\shared var lib.lvlib\\set encoder wheel"(FALSE ("rod up shared")) -> ()  [unwired: 1 in, 1 out]
        n429 = shared-variable ".\\local SCA shared var lib.lvlib\\SCA state control"(SCA_states."initialize" ("SC2 state")) -> ()  [unwired: 1 in, 1 out]
      }
    }
  }
  n430 = while {
    stop <- FALSE stop-if-true
    n431 = Wait Until Next ms Multiple(millisecond multiple=u32 50) -> ()  [unwired: 1 out]
  }
  n432 = disable-structure shown="Disabled" {
    frame Disabled {
      (unwired) 2794.0 ("y")
      (unwired) 2730.0 ("y")
      (unwired) 2613.0 ("y")
      (unwired) u32 16838 ("x")
      # "had been in check position case"
    }
    frame Enabled {
    }
  }
